vi "Text control 2 v5.3_pump-specific.vi"() -> ()   [LabVIEW 2016]
panel:
  in  "Tab Control":enum32{"Main", "Other parameters"}(tab)
  out "Line running":i32
  out "Total lines":i32
  out "Path":path=path "C:/users/rlp38/09Apr2009LTtesting/test2.txt"
  out "I vs Vg":cluster{"Y data in":dbl[], "X data in":dbl[]}[](graph)
  out "Is max":dbl format="%.2e"
  out "Id max":dbl format="%.2e"
  out "Ig max":dbl format="%.2e"
  out "Imax vs time":cluster{"Y data in":dbl[], "X data in":dbl[]}[](graph)
  out "Imin vs time":cluster{"Y data in":dbl[], "X data in":dbl[]}[](graph)
  out "I vs Vd":cluster{"Y data in":dbl[], "X data in":dbl[]}[](graph)
  in  "Script":string="#-------------------------------------------------------\n# Priming script\n#\n# Version 0.7\n# Author: Dimitrios Simatos\n# Last updated: 2017-10-22\n#-------------------------------------------------------\n# Description\n#\n# This script is designed to prime inlet ports 3, 5 and outlet port 2.\n#-------------------------------------------------------\n# Changes\n#\n# Changed drawing flow to 100 pulses/second.\n#-------------------------------------------------------\n# Important points\n#\n# Never leave any liquid in the pump to dry after the experiments. If they dry, the residue may block the valve.\n# Always run the cleaning cycle after the experiments.\n# Use clockwise rotation when going up in valve port numbers and vice versa.\n#-------------------------------------------------------\n# Things to do before running the script\n#\n# Set time units to minutes.\n# Set filenames.\n# Replace the tubing, if necessary.\n#-------------------------------------------------------\n# Port connections\n#\n# Port 1: Waste\n# Port 2: Waste\n# Port 3: Ultrapure water\n# Port 4: Nothing\n# Port 5: Phosphate buffer (pH=3.2 - 50 mM)\n# Port 6: Nothing\n#-------------------------------------------------------\n# Pumping cycles and execution time\n#\n# Execution time: 4 x 2 = 8 minutes\n# Ultrapure water must be the last to be pumped through the valve, to wash away residual ions.\n# There are 4 pumping cycles. The first two are small, priming cycles, and the last two are large, cleaning and priming cycles.\n# Each small pumping cycle primes the tubing of each port.\n# The last two cycle prime the tubing of the port containing ultrapure water (port 3) and also pump it through the valve, to clean the valve, the syringe, and prime the tubing of the device port (port 2).\n# The device must be disconnected from the port during the priming procedure.\n#-------------------------------------------------------\n# Volume of liquid needed\n#\n# Volume of liquid needed per small cycle: 200 ul\n# Volume of liquid needed per large cycle: 800 ul\n# Total volume of liquid needed per script run:\n# 200 ul of phosphate buffer (pH=3.2 - 50 mM)\n# 200 + 2 x 800 = 1800 ul of ultrapure water\n#-------------------------------------------------------\n# Parameters\n#\n# Syringe size: 1 ml\n# Step resolution N = 0.01 mm\n# Drawing flow V = 100 pulses/second (2000 ul/min)\n# Pumping flow V = 100 pulses/second (2000 ul/min)\n#-------------------------------------------------------\n# Cycle 1: Priming the tubing of port 5\npump /1ZR #initialize pump\npump /1Q #query pump\npump /1? #report absolute plunger position\n#pump /1?6 #report valve position\nwait-min 1 #wait 1 minute\npump /1N0R #set step resolution: 0.01 mm\npump /1Q #query pump\npump /1? #report absolute plunger position (the plunger should be at 0)\npump /1?6 #report valve position\nwait 1000 #wait 1 second\npump /1V100R #choose speed: 100 steps/s (200 ul/min)\npump /1Q #query pump\nwait 1000 #wait 1 second\npump /1O5R #go to port 5, counterclockwise rotation\npump /1Q #query pump\npump /1?6 #report valve position\nwait 1000 #wait 1 second\npump /1A600R #go to absolute position 600 (= draw 200 ul)\n# The position of the plunger depends on the volume of the tubing. The syringe must draw enough liquid to fill the tubing.\nwait 30000 #wait 30 seconds\npump /1Q #query pump\npump /1? #report absolute plunger position (the plunger should have finished moving)\n#pump /1?6 #report valve position\npump /1I1R #switch to port 1, clockwise rotation\npump /1Q #query pump\npump /1?6 #report valve position\npump /1A0R #go to absolute position 0 (= empty syringe)\npump /1Q #query pump\npump /1? #report absolute plunger position (the plunger should be moving to 0)\n#pump /1?6 #report valve position\nwait-min 1 #wait 1 minute\n#-------------------------------------------------------\n# Cycle 2: Priming the tubing of port 3\n#pump /1ZR #initialize pump\npump /1Q #query pump\npump /1? #report absolute plunger position\npump /1?6 #report valve position\nwait-min 1 #wait 1 minute\npump /1N0R #set step resolution: 0.01 mm\npump /1Q #query pump\npump /1? #report absolute plunger position (the plunger should be at 0)\npump /1?6 #report valve position\nwait 1000 #wait 1 second\npump /1V100R #choose speed: 100 steps/s (200 ul/min)\npump /1Q #query pump\nwait 1000 #wait 1 second\npump /1I3R #go to port 3, clockwise rotation\npump /1Q #query pump\npump /1?6 #report valve position\nwait 1000 #wait 1 second\npump /1A600R #go to absolute position 600 (= draw 200 ul)\n# The position of the plunger depends on the volume of the tubing. The syringe must draw enough liquid to fill the tubing.\nwait 30000 #wait 30 seconds\npump /1Q #query pump\npump /1? #report absolute plunger position (the plunger should have finished moving)\n#pump /1?6 #report valve position\npump /1O1R #switch to port 1, counterclockwise rotation\npump /1Q #query pump\npump /1?6 #report valve position\npump /1A0R #go to absolute position 0 (= empty syringe)\npump /1Q #query pump\npump /1?6 #report valve position\npump /1? #report absolute plunger position (the plunger should be moving to 0)\n#pump /1?6 #report valve position\nwait-min 1 #wait 1 minute\n#-------------------------------------------------------\n# Cycle 3: Cleaning the syringe and the tubing of port 2 (1/2)\n#pump /1ZR #initialize pump\npump /1Q #query pump\npump /1? #report absolute plunger position\npump /1?6 #report valve position\nwait-min 1 #wait 1 minute\npump /1N0R #set step resolution: 0.01 mm\npump /1Q #query pump\npump /1? #report absolute plunger position (the plunger should be at 0)\npump /1?6 #report valve position\nwait 1000 #wait 1 second\npump /1V100R #choose speed: 100 steps/s (200 ul/min)\npump /1Q #query pump\nwait 1000 #wait 1 second\npump /1I3R #go to port 3, clockwise rotation\npump /1Q #query pump\npump /1?6 #report valve position\nwait 1000 #wait 1 second\npump /1A2400R #go to absolute position 2400 (= draw 800 ul)\n# The position of the plunger depends on the volume of the tubing. The syringe must draw enough liquid to fill the tubing.\nwait 30000 #wait 30 seconds\npump /1Q #query pump\npump /1? #report absolute plunger position (the plunger should have finished moving)\n#pump /1?6 #report valve position\npump /1O2R #switch to port 2, counterclockwise rotation\npump /1Q #query pump\npump /1?6 #report valve position\npump /1A0R #go to absolute position 0 (= empty syringe)\npump /1Q #query pump\npump /1? #report absolute plunger position (the plunger should be moving to 0)\n#pump /1?6 #report valve position\nwait-min 1 #wait 1 minute\n#-------------------------------------------------------\n# Cycle 4: Cleaning the syringe and the tubing of port 2 (2/2)\n#pump /1ZR #initialize pump\npump /1Q #query pump\npump /1? #report absolute plunger position\npump /1?6 #report valve position\nwait-min 1 #wait 1 minute\npump /1N0R #set step resolution: 0.01 mm\npump /1Q #query pump\npump /1? #report absolute plunger position (the plunger should be at 0)\npump /1?6 #report valve position\nwait 1000 #wait 1 second\npump /1V100R #choose speed: 100 steps/s (200 ul/min)\npump /1Q #query pump\nwait 1000 #wait 1 second\npump /1I3R #go to port 3, clockwise rotation\npump /1Q #query pump\npump /1?6 #report valve position\nwait 1000 #wait 1 second\npump /1A2400R #go to absolute position 2400 (= draw 800 ul)\n# The position of the plunger depends on the volume of the tubing. The syringe must draw enough liquid to fill the tubing.\nwait 30000 #wait 30 seconds\npump /1Q #query pump\npump /1? #report absolute plunger position (the plunger should have finished moving)\n#pump /1?6 #report valve position\npump /1O2R #switch to port 2, counterclockwise rotation\npump /1Q #query pump\npump /1?6 #report valve position\npump /1A0R #go to absolute position 0 (= empty syringe)\npump /1Q #query pump\npump /1? #report absolute plunger position (the plunger should be moving to 0)\n#pump /1?6 #report valve position\nwait-min 1 #wait 1 minute\n#-------------------------------------------------------"
  out "Command running:":string
  out "Serial port data":string
  out "Elapsed Time":dbl caption="Elapsed Time (s)"
  in  "Units":u16(ring)=1 items=["Seconds", "Minutes", "Hours"]
  in  "Time Offset":dbl caption="Set Start Time (s)"
  in  "Reset":bool
  in  "Auto Reset":bool
  in  "integration time":u32(slide) max=2 step=1 scale=0.0..2.0
  in  "Interrupt run":bool
  out "Absolute plunger position vs time":cluster{"Y data in":dbl[], "X data in":dbl[]}[](graph)
  out "Valve position vs time":cluster{"Y data in":dbl[], "X data in":dbl[]}[](graph)
  in  "Halt pump":bool
  in  "Hard stop pump":bool
  out "Is on":dbl format="%.2e"
  out "Id on":dbl format="%.2e"
  out "Ig on":dbl format="%.2e"
  out "Ion vs time":cluster{"Y data in":dbl[], "X data in":dbl[]}[](graph)
  out "Ioff vs time":cluster{"Y data in":dbl[], "X data in":dbl[]}[](graph)
  out "Ig min":dbl format="%.2e"
  out "Id min":dbl format="%.2e"
  out "Is min":dbl format="%.2e"
  out "Is off":dbl format="%.2e"
  out "Id off":dbl format="%.2e"
  out "Ig off":dbl format="%.2e"
  in  "Gate Range\nmode":u16(ring) items=["Auto", "Limited", "Fixed"]
  in  "Gate Range":u8(slide)=6 max=11 scale=0.0..11.0
  in  "Source/Drain\nRange mode":u16(ring) items=["Auto", "Limited", "Fixed"]
  in  "Source/Drain Range":u8(slide)=6 max=11 scale=0.0..11.0
  in  "Panel Controls":T1={"Emergency Stop"=refnum, "TransGraph Max"=1e-05, "Text/Graph (text=false)"=TRUE} {"TransGraph Max" format="%.2e"}
  in  "Panel Controls 2":T2={"Emergency Stop"=refnum, "TransGraph Max"=1e-05, "Text/Graph (text=false)"=TRUE, "TransGraph Min"=1e-11} {"TransGraph Min" format="%.2e"; "TransGraph Max" format="%.2e"}
  in  "SMU4":cluster{"on/off":bool, "Voltage":dbl} {"Voltage" min=-100.0 max=100.0 format="%.2f"}
  in  "Full Reset":bool
  in  "Standby":T3
  out "error out":errorcluster
  in  "Delay before read (ms)":u32=1000
  in  "byte count":u32=64
  in  "Serial End Mode for Reads":u16(ring)=2 items=["None", "LastBit", "TermChar"]
  in  "Timeout (ms)":u32=10000
  in  "Enable Termination\nChar (T)":bool=TRUE
  in  "Termination char\n(0xA = '\\n' = LF)\n(0xD = '\\r' = CR)":u8=13 format="%.0x"
  in  "flow control":u16(ring) items=["None"=0, "XON/XOFF"=1, "RTS/CTS"=2, "DTR/DSR"=4]
  in  "stop bits":u16(ring)=10 items=["1.0"=10, "1.5"=15, "2.0"=20]
  in  "parity":u16(ring) items=["None", "Odd", "Even", "Mark", "Space"]
  in  "data bits":u16=8 min=5 max=8 step=1
  in  "VISA resource name":refnum<visa-resource-name>="COM6"
  in  "baud rate":u32=9600
  in  "Drain: Compliance":dbl=0.001 format="%.8f"
  in  "Gate: Compliance":dbl=0.001 format="%.8f"
  in  "hold time /s":dbl format="%.2f"
  in  "delay time /s":dbl format="%.2f"
  in  "Integration time (short)":dbl=0.0019 min=8e-05 max=0.0019 step=8e-05 format="%^.0e"
  in  "Integration time (long)":dbl=0.32 min=0.04 max=2.0 step=0.02 format="%.2f"
  in  "Step delay /s":dbl format="%.2f"
  in  "Filename (variable part)":string="step_1_ultrapure_H2O_"
  in  "Suffix (script)":string="step_1_ultrapure_H2O_script.txt"
  in  "Gate":T4={"Gate Start"=0.0, "Gate Stop"=2.0, "Gate Step (linear only)"=1.0, "Gate Compliance"=0.0001, "Gate PComp"=0.0, "Range mode"=0, "Range"=6} {"Range" max=11 scale=0.0..11.0; "Range mode" items=["Auto", "Limited", "Fixed"]; "Gate PComp" format="%^.2e"; "Gate Compliance" format="%^.2e"; "Gate Step (linear only)" format="%^.4e"; "Gate Stop" format="%^.4e"; "Gate Start" format="%^.4e"}
  in  "Drain 2":T5={"Drain Start"=0.0, "Drain Stop"=2.0, "Drain Compliance"=0.0001, "Drain Step"=1.0, "Drain PComp"=0.0, "Range mode"=0, "Range"=6} {"Range" max=11 scale=0.0..11.0; "Range mode" items=["Auto", "Limited", "Fixed"]; "Drain PComp" format="%^.2e"; "Drain Step" format="%^.4e"; "Drain Compliance" format="%^.2e"; "Drain Stop" format="%^.4e"; "Drain Start" format="%^.4e"}
  in  "Timings 2":T6={"integration time"=0, "Short/Long integration time"=0.00064, "hold time (sec)"=0.0, "delay time (sec)"=0.0, "Step Time (0 disables)"=0.0, "sweep method"=0, "Pulse period"=0.005, "Base voltage"=0.0, "Pulse width"=0.0005} {"Pulse width" min=0.0005 max=0.1 step=0.0001 format="%.4f"; "Base voltage" format="%^.4e"; "Pulse period" min=0.005 max=1.0 step=0.0001 format="%.4f"; "sweep method" items=["Continuous", "Pulsed"]; "Step Time (0 disables)" format="%.2f"; "delay time (sec)" format="%.4f"; "hold time (sec)" format="%.4f"; "Short/Long integration time" format="%^.0e"; "integration time" scale=0.0..2.0}
  # "Syntax:\nitime [s|m|l]\ngaterangemode [a|l|f]\ndrainrangemode [a|l|f]\npulsed [on|off] PulsePeriod(sec) PulseBaseVoltage PulseONWidth(sec)\nstandby [on l off]\nwait NumMilliseconds\nwait-min NumMinutes\n# texthere = comment\ntransfer [s|d] VgStart VgStop VgStep VdStart VdStop VdStep\noutput [s|d] VgStart VgStop VgStep VdStart VdStop VdStep\nsample Vg Vd NumSamples Time(s) SampleInterval(s)\nsamplei Idg NumSamples Time(s) SampleInterval(s) VDGcompliance\n100 samples is approximately 13 seconds with medium integration\n# if in doubt use SampleInterval(s) = 0.004\nstressV VG VD IGcompliance IDcompliance Duration(sec)\nstressI IDG VDGcompliance Duration(sec)\nvsu2pulse Bias Duration(s)\npulsedstressV [s|d] VEstop VgON VgOFF Period(s) PulseONwidth(s) Vd\nsample-fpp Vg Vd NumSamples Time\nresample-fpp Vg Vd\ntransfer-fpp [s|d] VgStart VgStop VgStep VdStart VdStop VdStep\noutput-fpp [s|d] VgStart VgStop VgStep VdStart VdStop VdStep\nserial SerialPortCommand\npump SerialPortCommand for the SPM pump\n\nSPM Pump Syntax (<x>: pump number, use 1 if only one pump):\nif the command syntax contains [R], then append the letter R to the command\n/<x>Q: query (a query command should follow each command)\n/<x>Z[R] or /<x>Y[R]: initialize pump\n/<x>N<n>[R] (<n>=0,1): <0> (<1>) microstep 0.01 mm (0.00125 mm) resolution\n/<x>I<n> (<n>=0-6): turn to port number n (clockwise)\n/<x>O<n> (<n>=0-6): turn to port number n (counterclockwise)\n/<x>X: Re-execute last command string\n/<x>G<n>[R] (<n>=0-60000): repeat command sequence (default: 0, 0=loop forever)\n/<x>g: Mark the start of a repeat sequence (max = 10)\n/<x>M<n>[R] (<n>=0-86400000): delay command execution by n milliseconds\n/<x>H: Halt; Pause the sequence after finishing the current move\n/<x>T: Hardstop; Interrupt the current move and suppress it from the sequence\n/<x>A<n>[R] (<n>=0-3000 with N=0, 0-24000 with N=1): absolute position\n/<x>P<n>[R] (<n>=0-3000 with N=0, 0-24000 with N=1): relative pickup\n/<x>D<n>[R] (<n>=0-3000 with N=0, 0-24000 with N=1): relative dispense\n/<x>V<n>[R] (<n>=1-1600 default: 150): set peak speed (pulses/sec)\nNOTE: The lowest speed limit is 1 pulse/sec, not 5, as the manual states.\n/<x>S<n>[R] (<n>=10-40 default: 22): set speed (NOT in pulses/sec, look in manual)\nNOTE: When controlled with absolute position, one does not need to pay special attention to the syringe that is mounted on the pump.\nWithdraw from lower stage (ports 3, 5), dispense from higher stage (ports 2, 4, 6).\nConnect Port 1 to waste."
  # "Time"
  # "1\n2\n3\n4\n5\n6\n7\n8\n9\n10\n11\n12\n13\n14\n15\n16\n17\n18\n19\n20"
  # "Serial port settings"
  # "Filename settings"
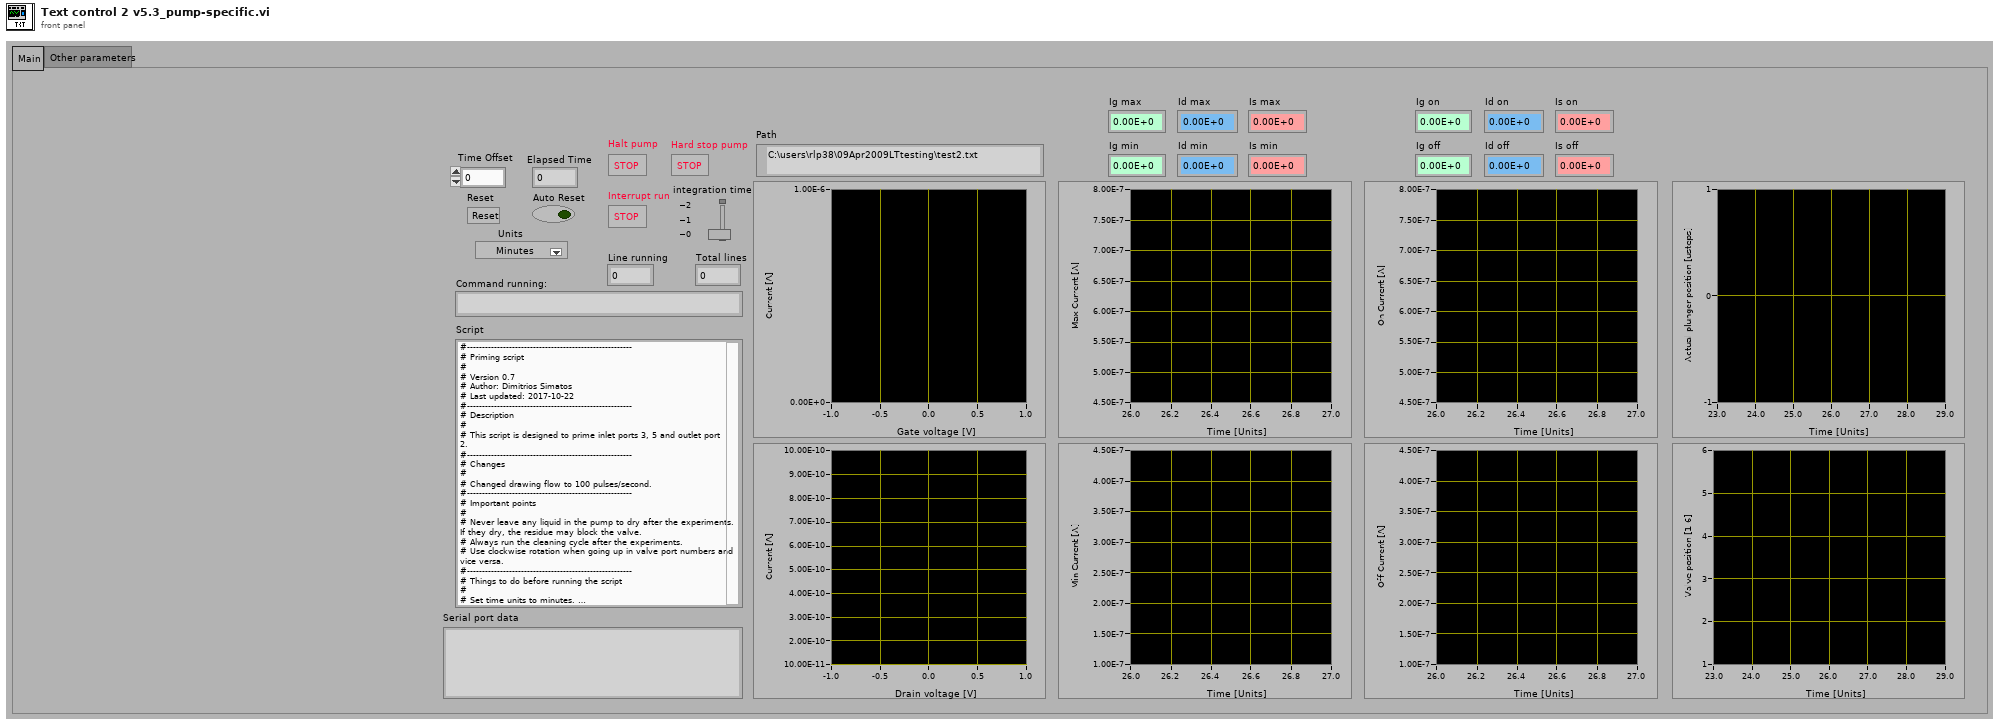
[diagram p1: front panel]
types:
  T1 = cluster{"Emergency Stop":refnum<vi>, "TransGraph Max":dbl, "Text/Graph (text=false)":bool}
  T2 = cluster{"Emergency Stop":refnum<vi>, "TransGraph Max":dbl, "Text/Graph (text=false)":bool, "TransGraph Min":dbl}
  T3 = cluster{"Gate Standby":bool, "Drain Standby":bool}
  T4 = cluster{"Gate Start":dbl, "Gate Stop":dbl, "Gate Step (linear only)":dbl, "Gate Compliance":dbl, "Gate PComp":dbl, "Range mode":u16, "Range":u8}
  T5 = cluster{"Drain Start":dbl, "Drain Stop":dbl, "Drain Compliance":dbl, "Drain Step":dbl, "Drain PComp":dbl, "Range mode":u16, "Range":u8}
  T6 = cluster{"integration time":u32, "Short/Long integration time":dbl, "hold time (sec)":dbl, "delay time (sec)":dbl, "Step Time (0 disables)":dbl, "sweep method":u16, "Pulse period":dbl, "Base voltage":dbl, "Pulse width":dbl}
  T7 = enum16{"open", "replace", "create", "open or create", "replace or create", "replace or create with confirmation"}
  T8 = cluster{"V2 Start":dbl, "V2 Step":dbl, "Number of points":i32}
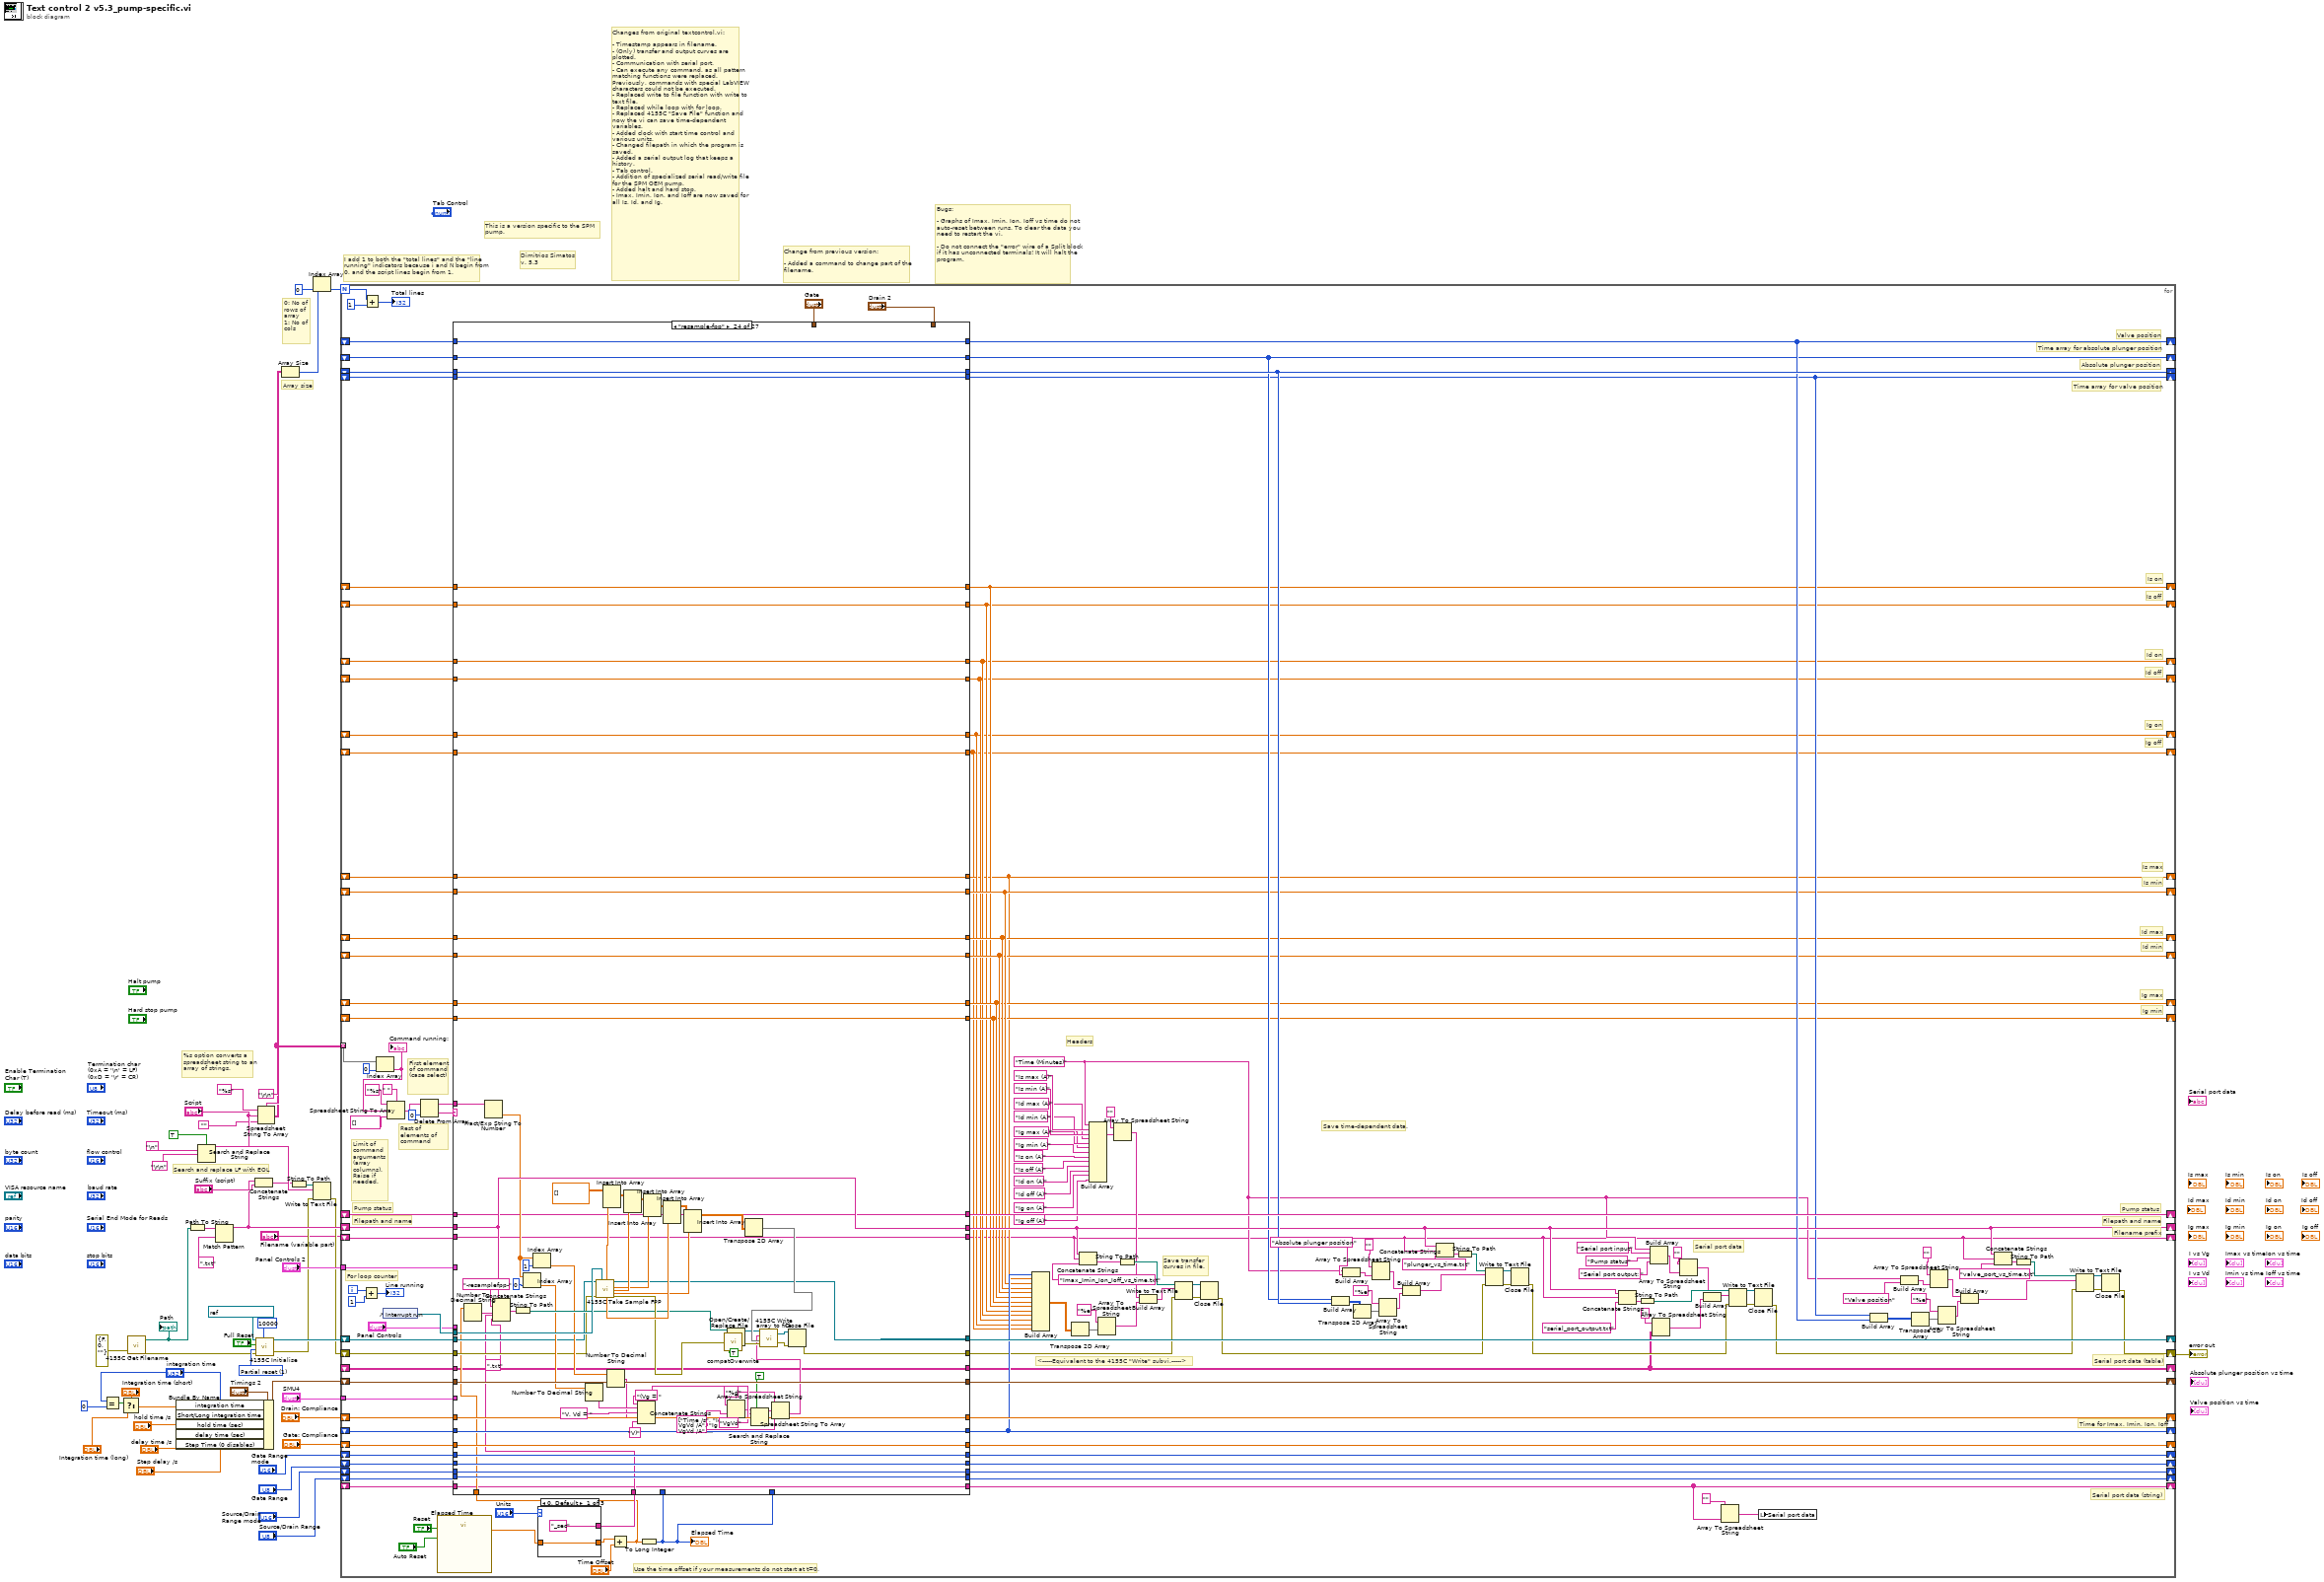
[diagram p0: block diagram]
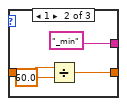
[diagram p2: hidden frame]
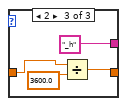
[diagram p3: hidden frame]
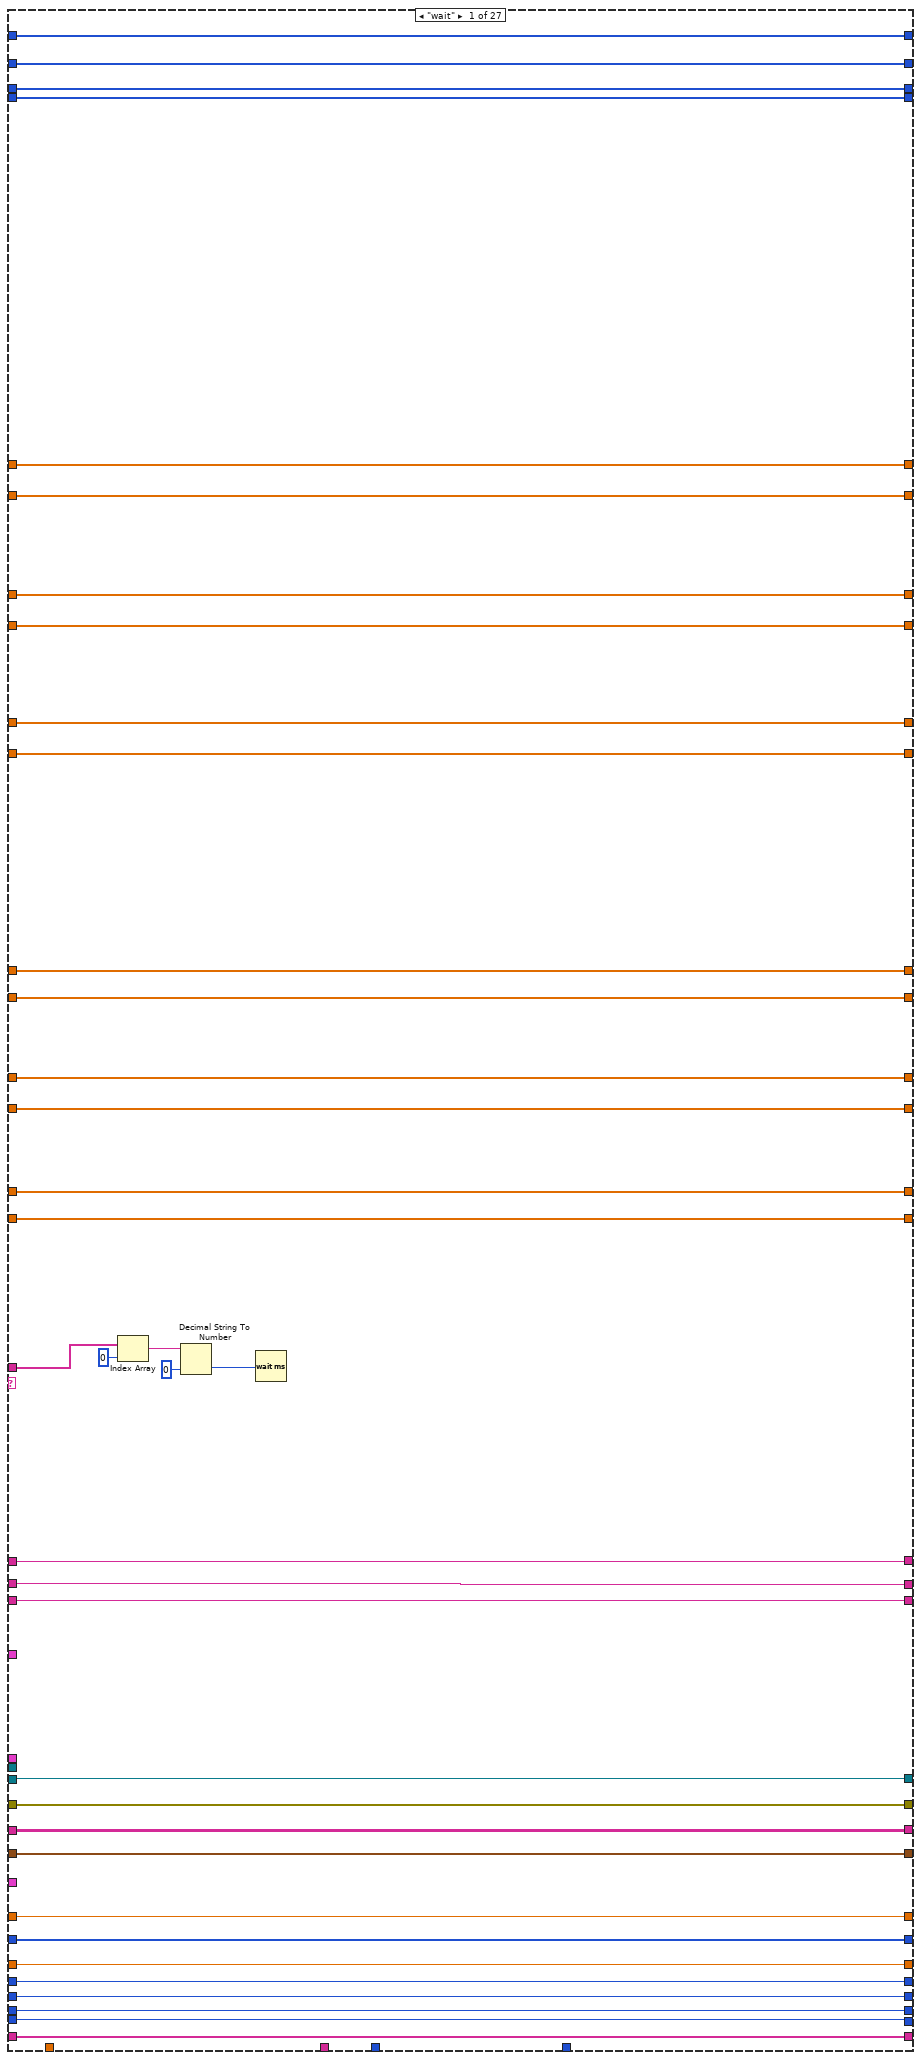
[diagram p4: hidden frame]
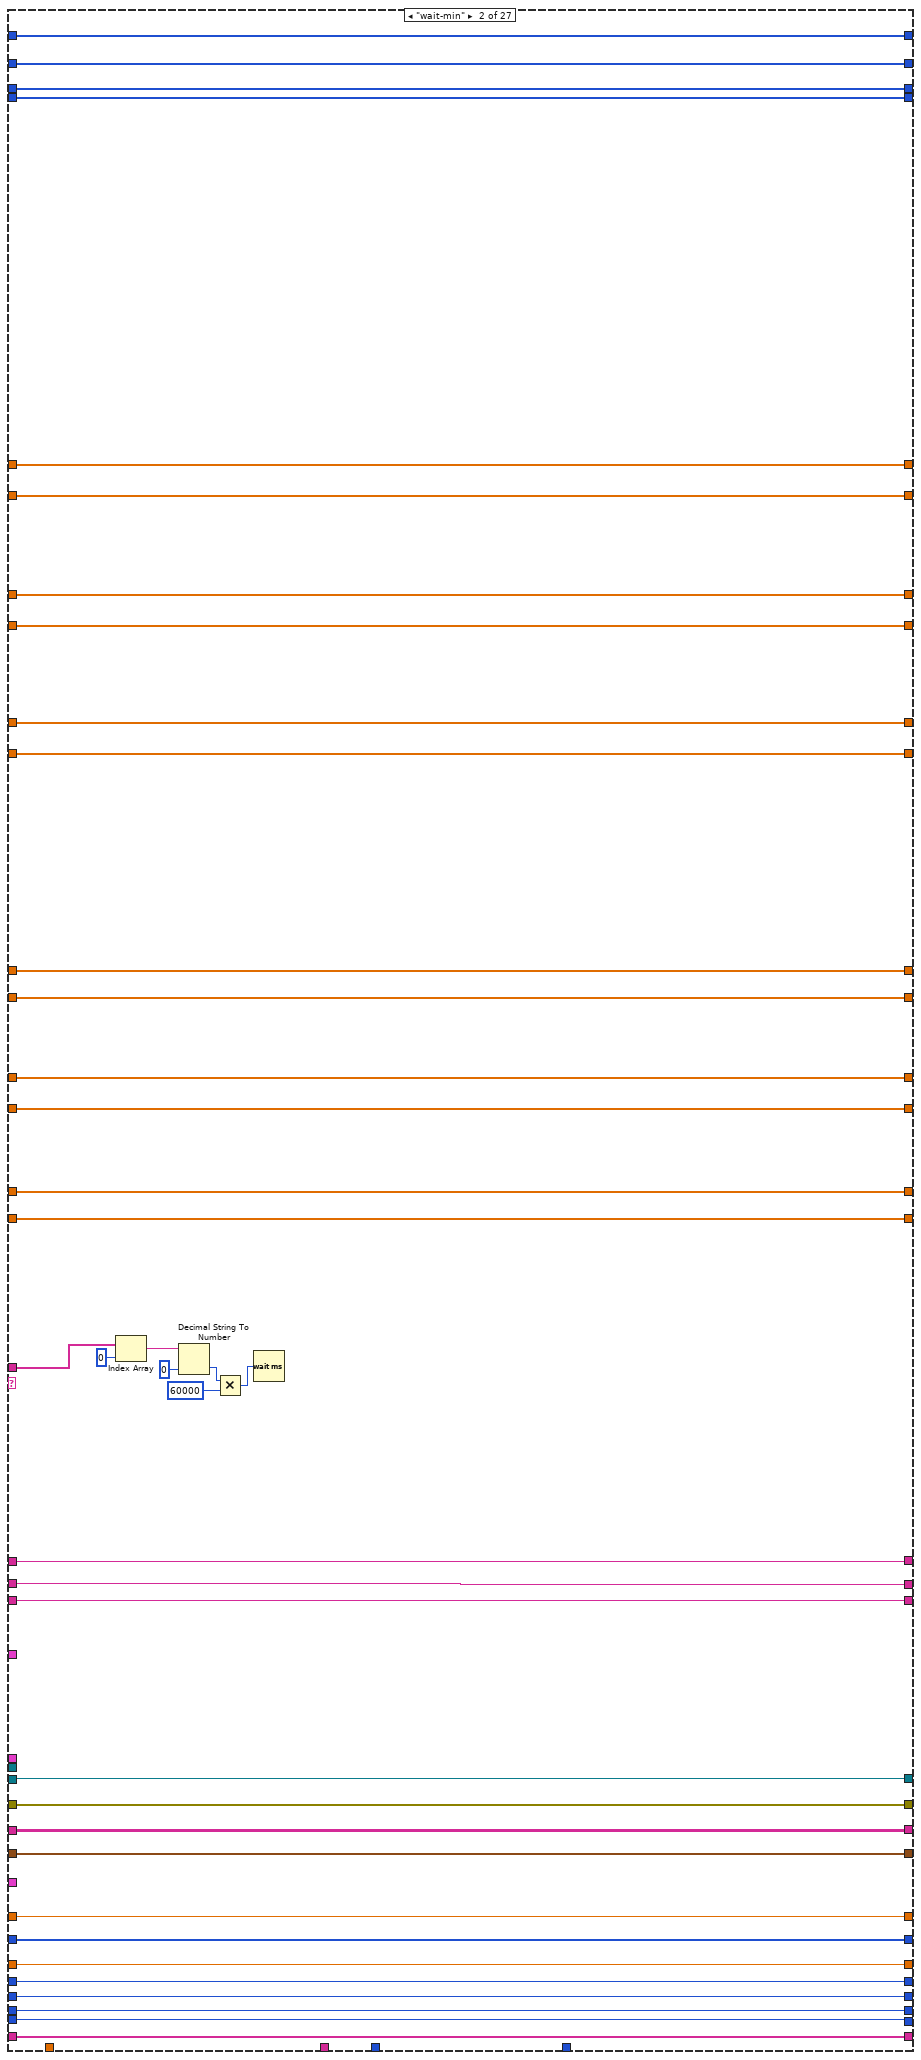
[diagram p5: hidden frame]
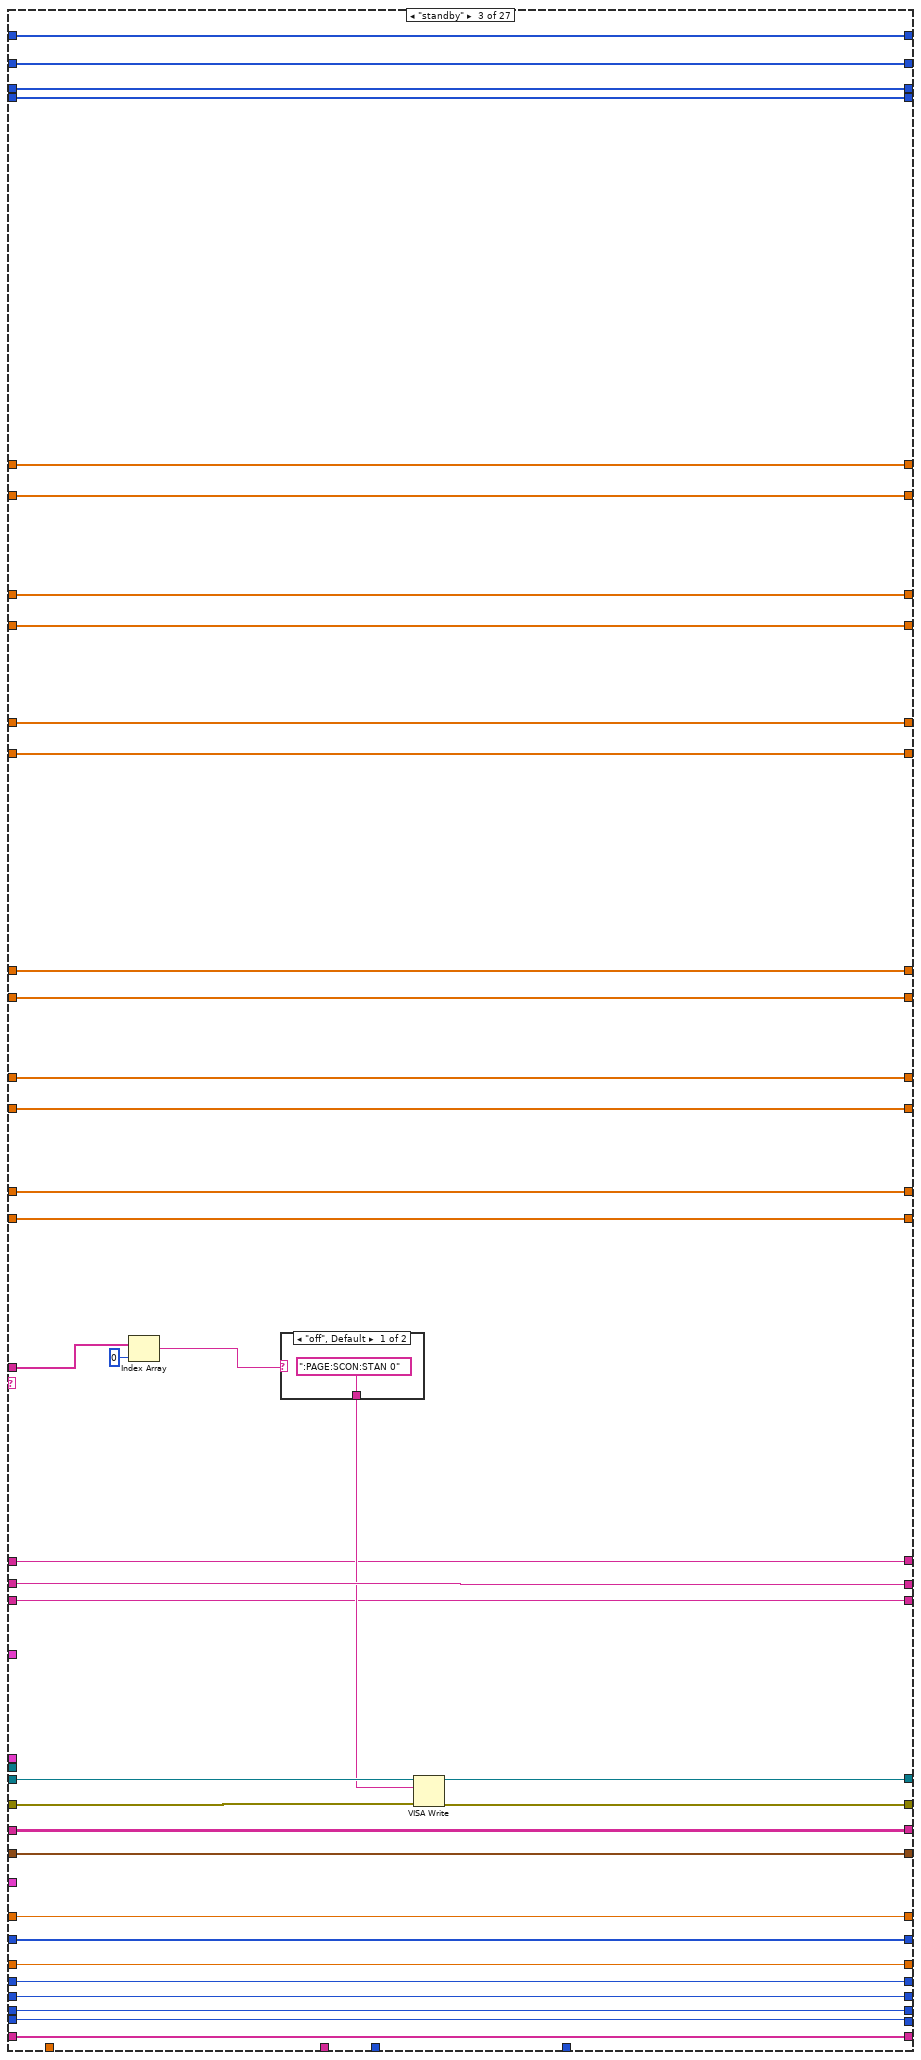
[diagram p6: hidden frame]
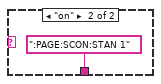
[diagram p7: hidden frame]
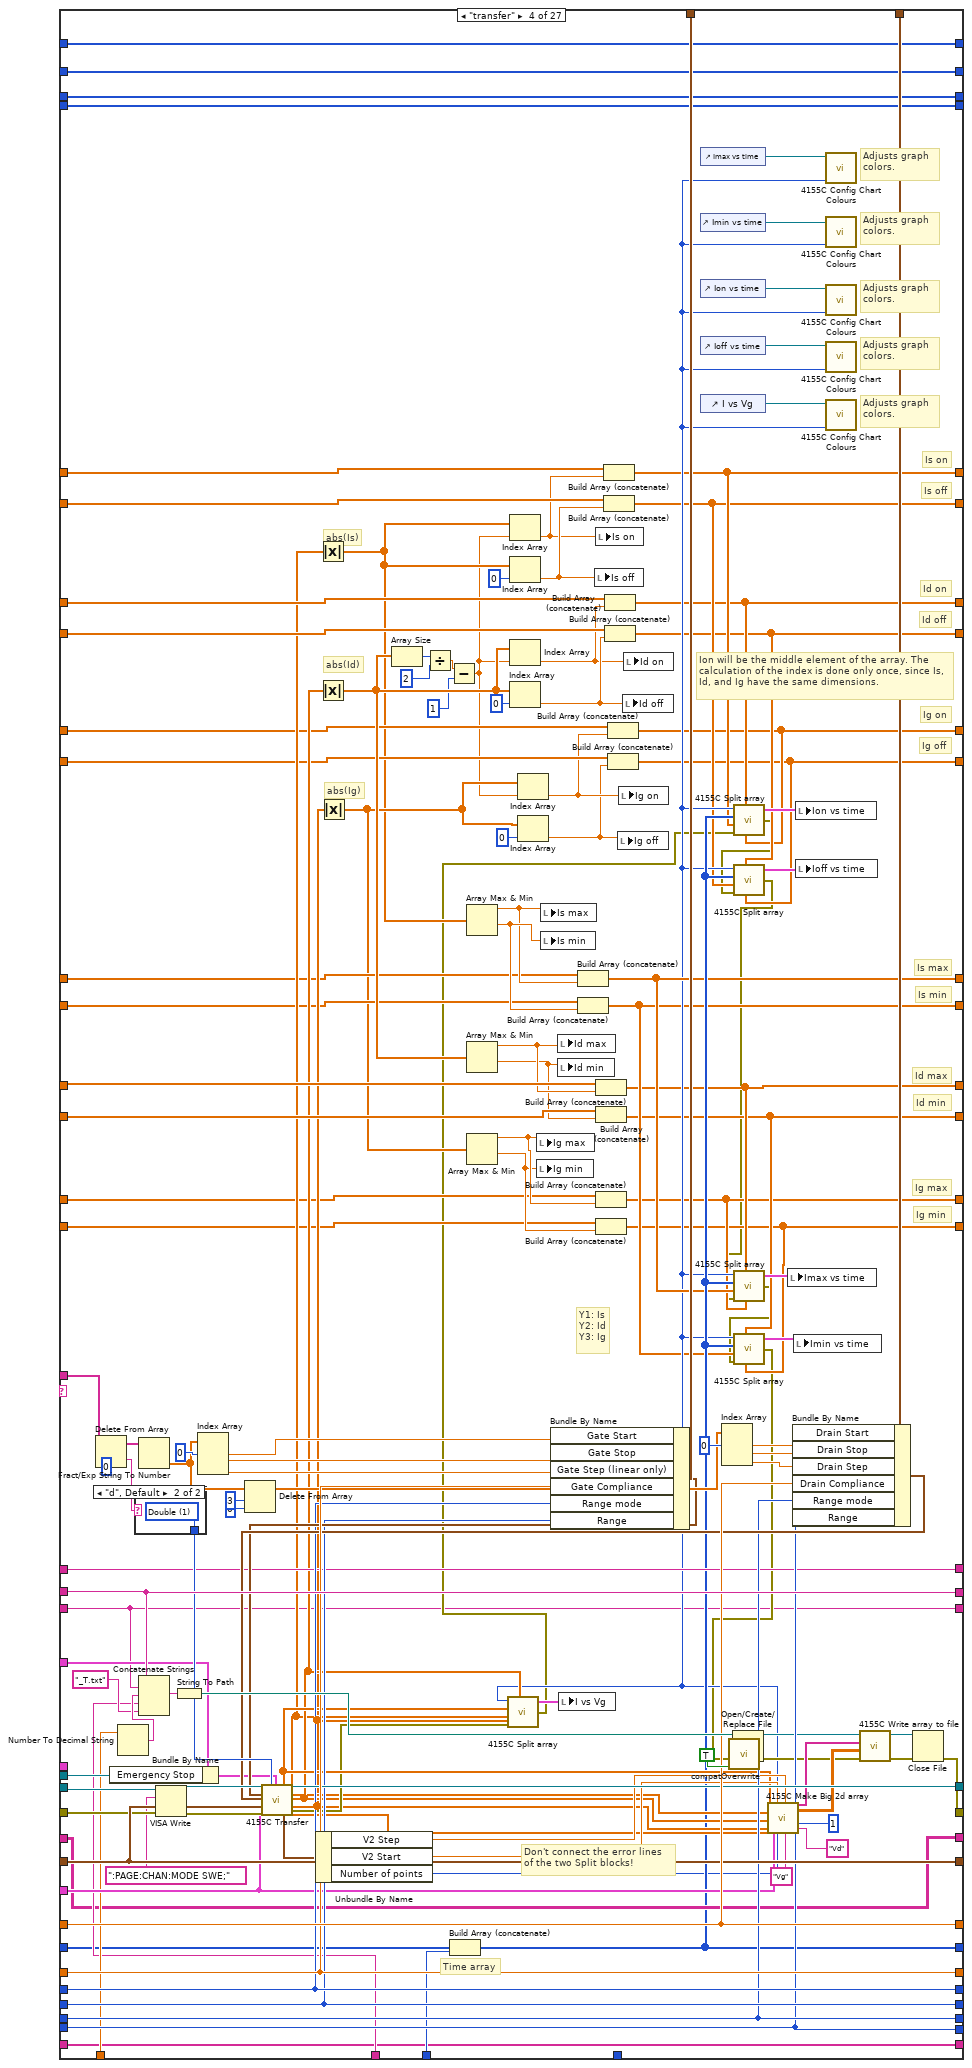
[diagram p8: hidden frame]
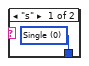
[diagram p9: hidden frame]
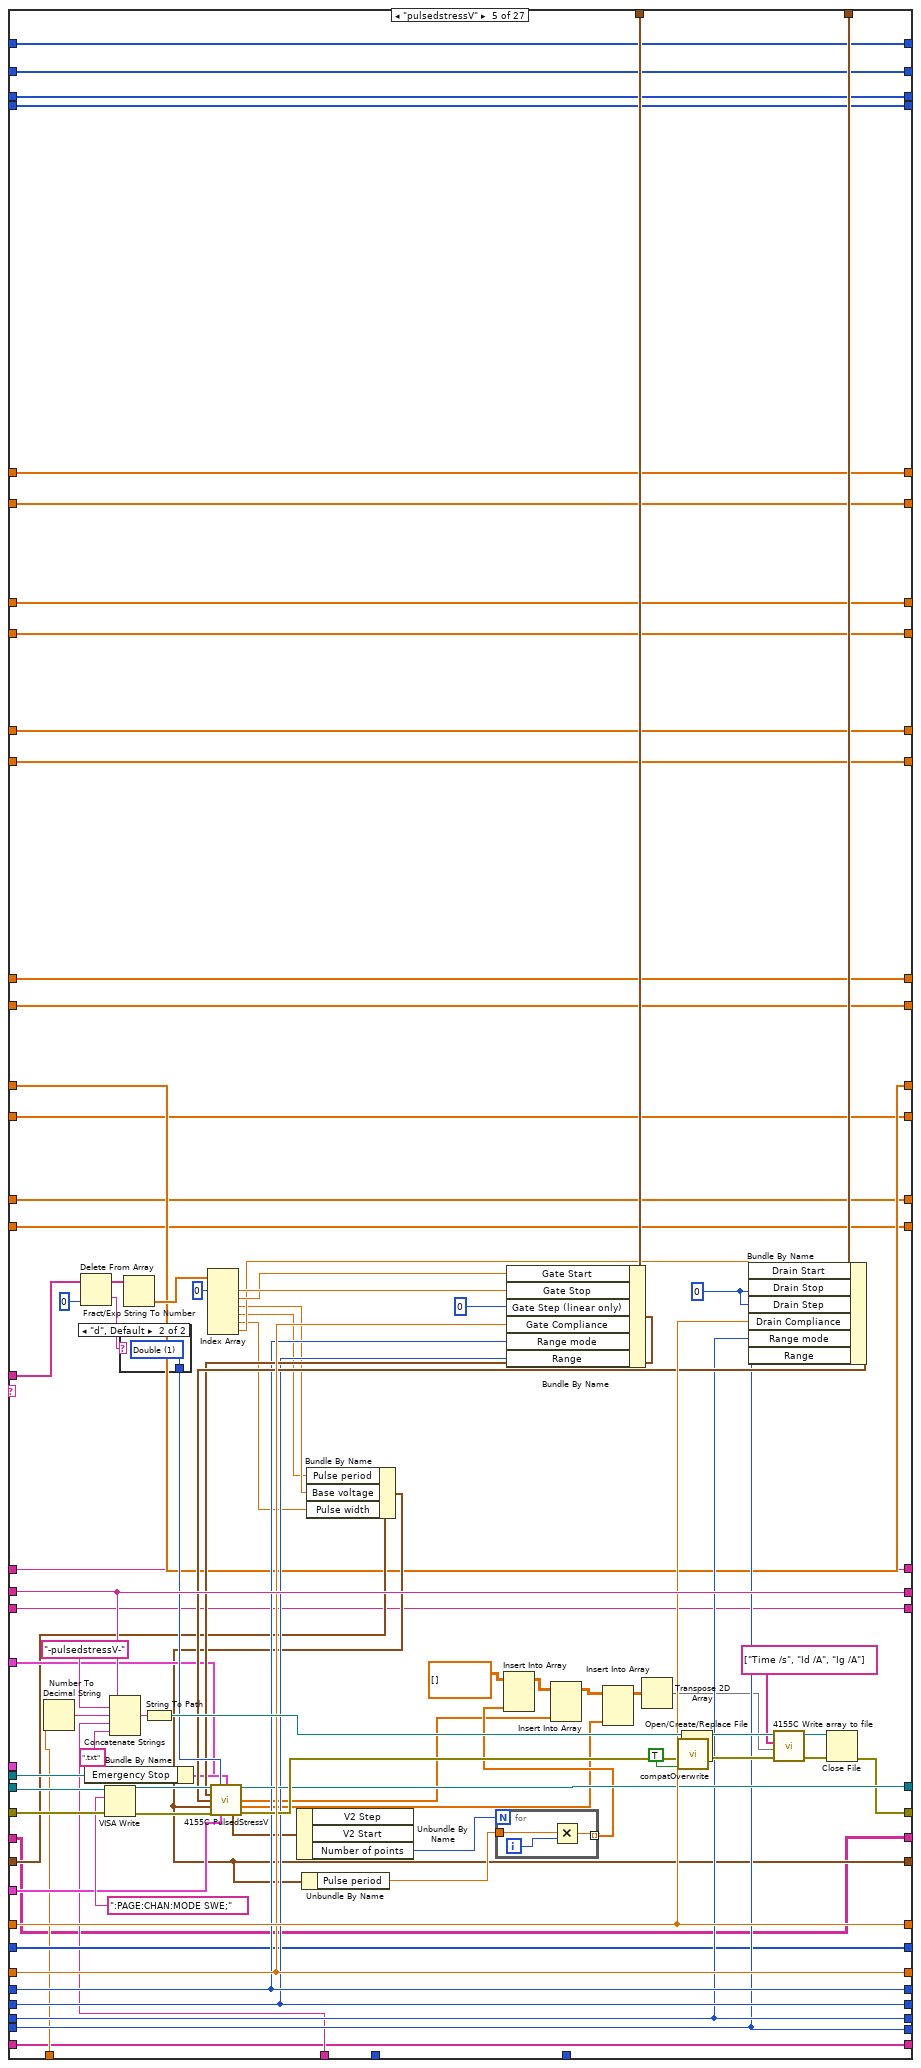
[diagram p10: hidden frame]
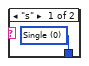
[diagram p11: hidden frame]
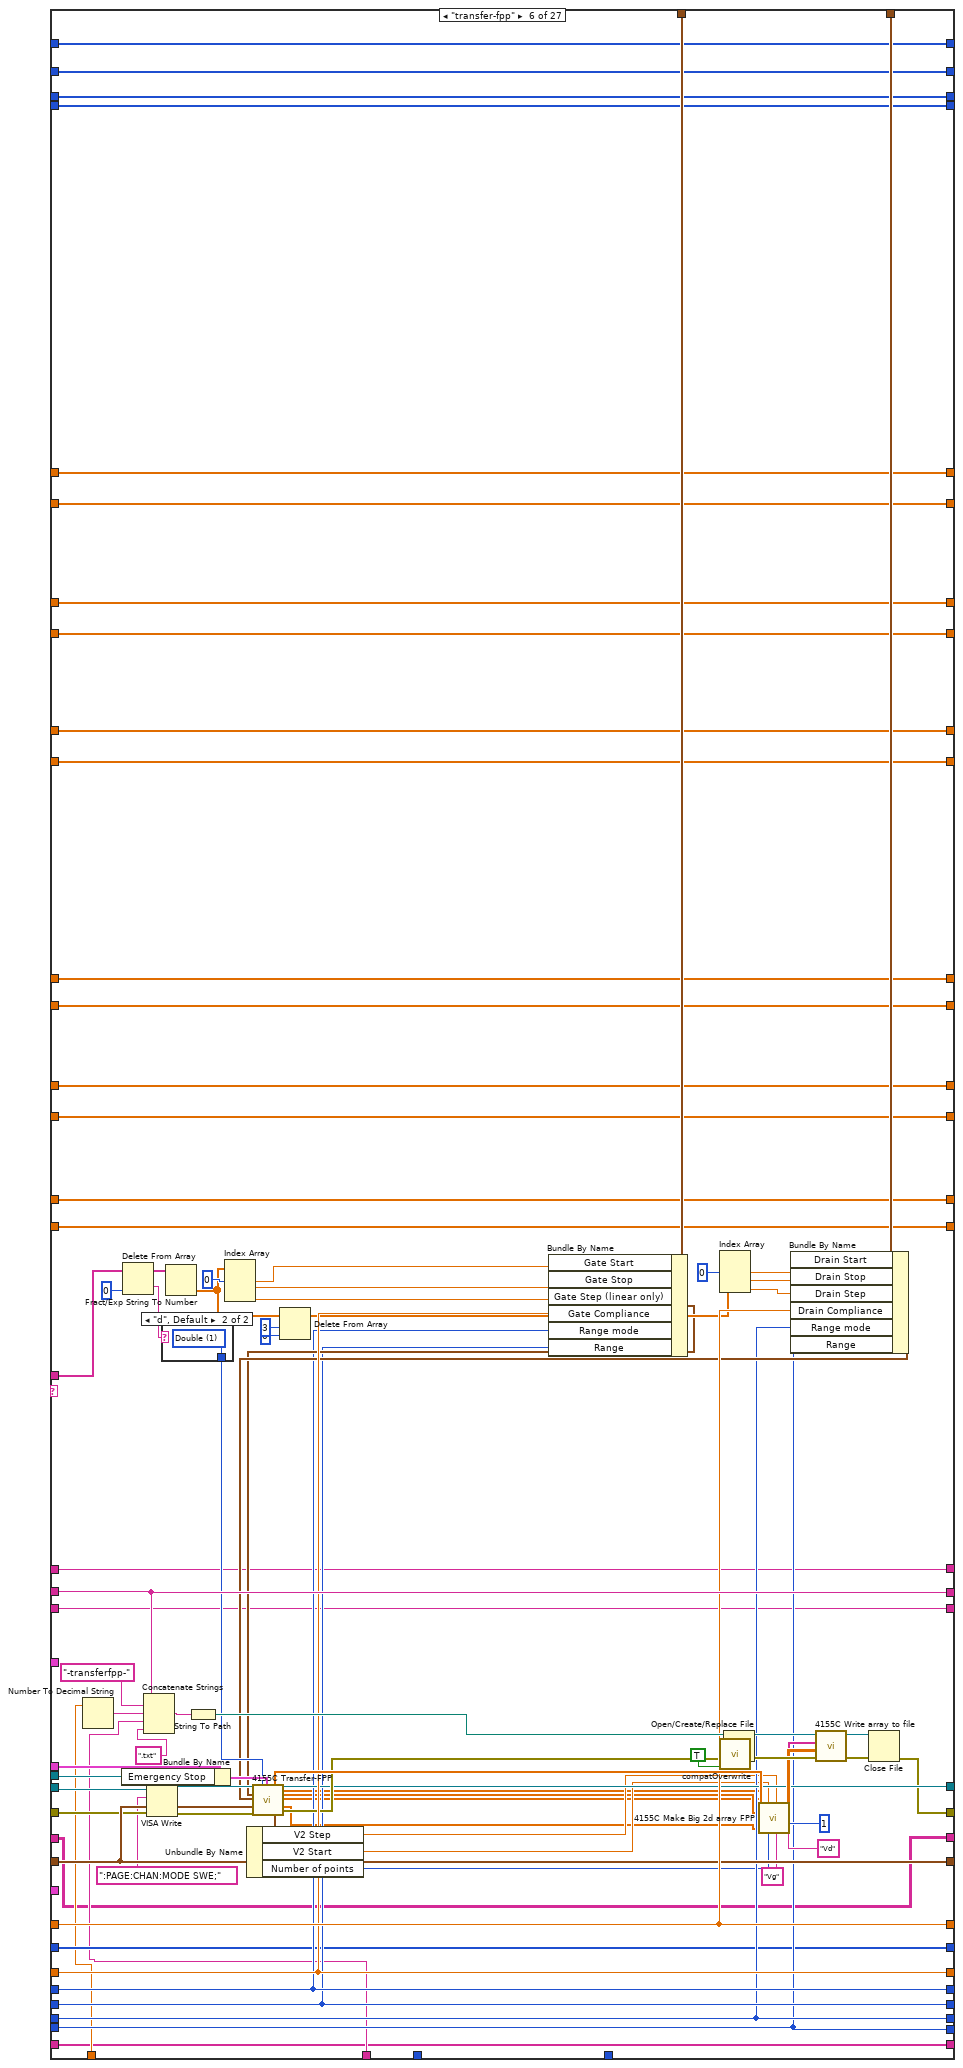
[diagram p12: hidden frame]
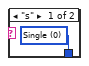
[diagram p13: hidden frame]
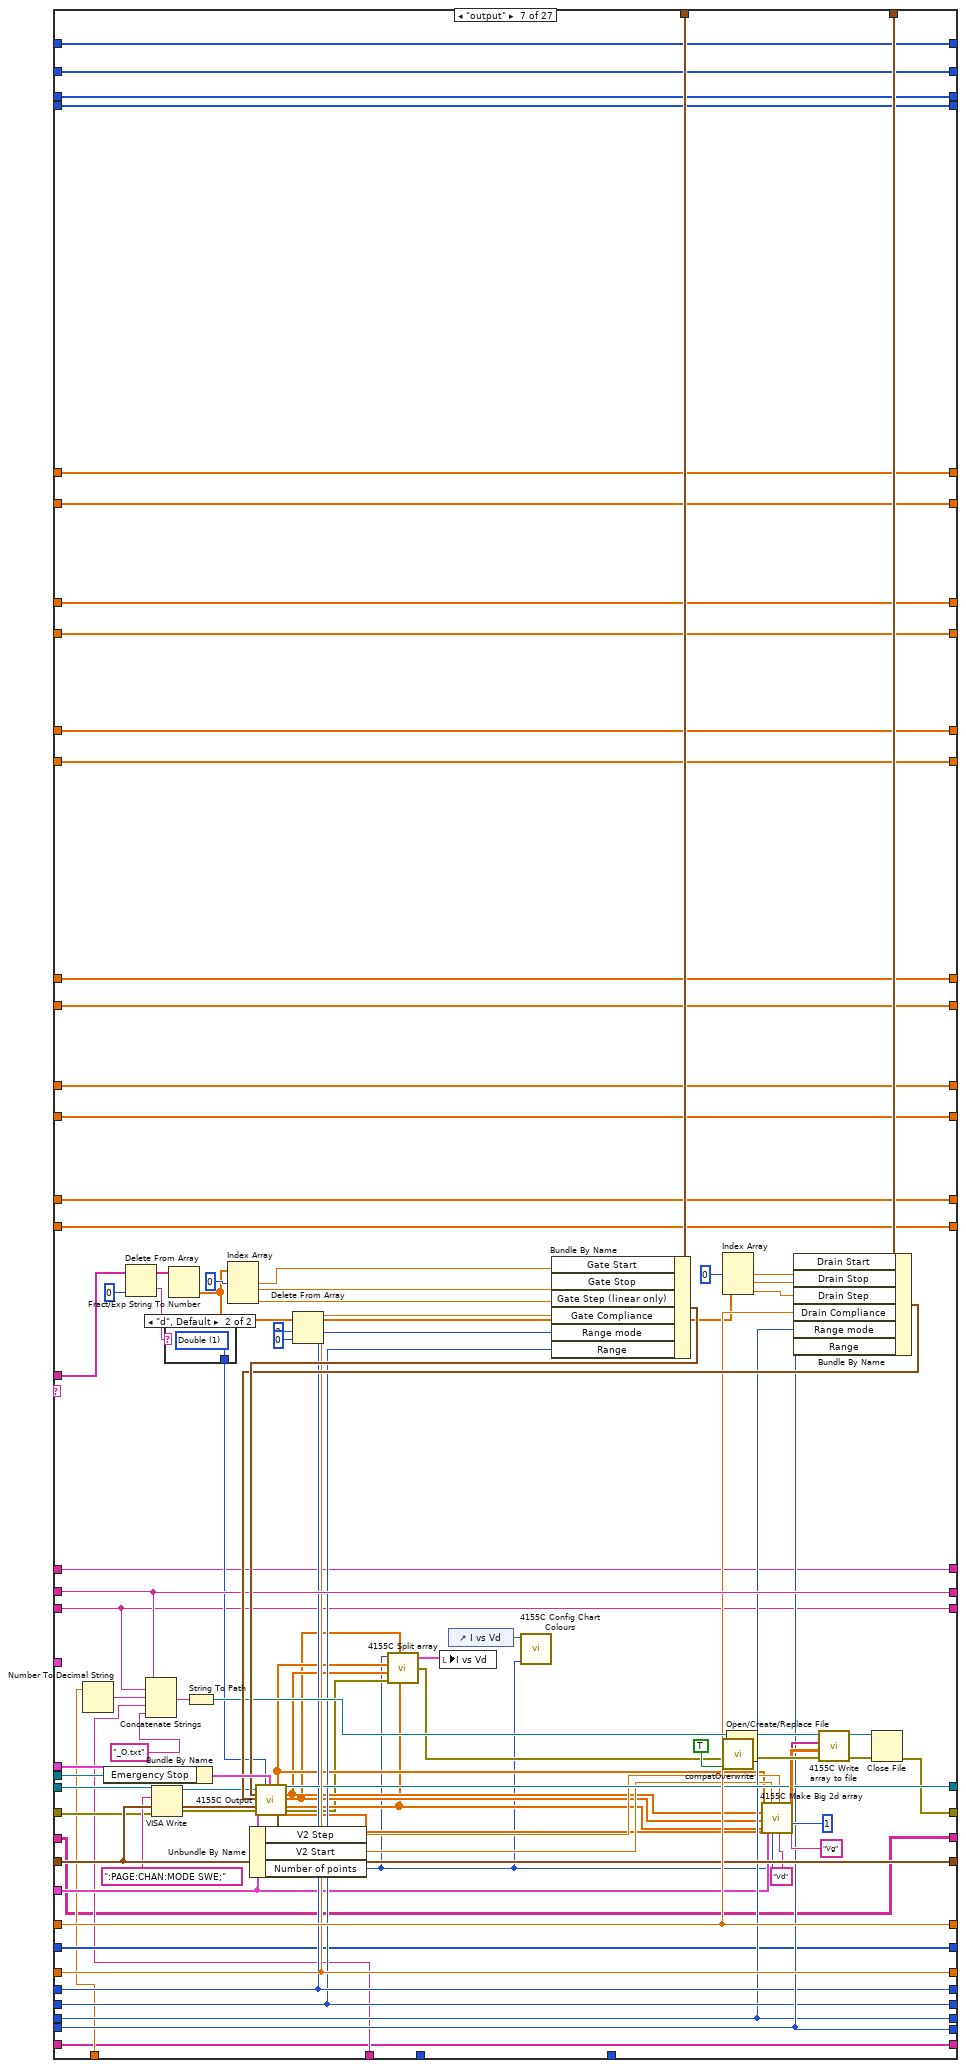
[diagram p14: hidden frame]
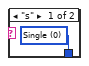
[diagram p15: hidden frame]
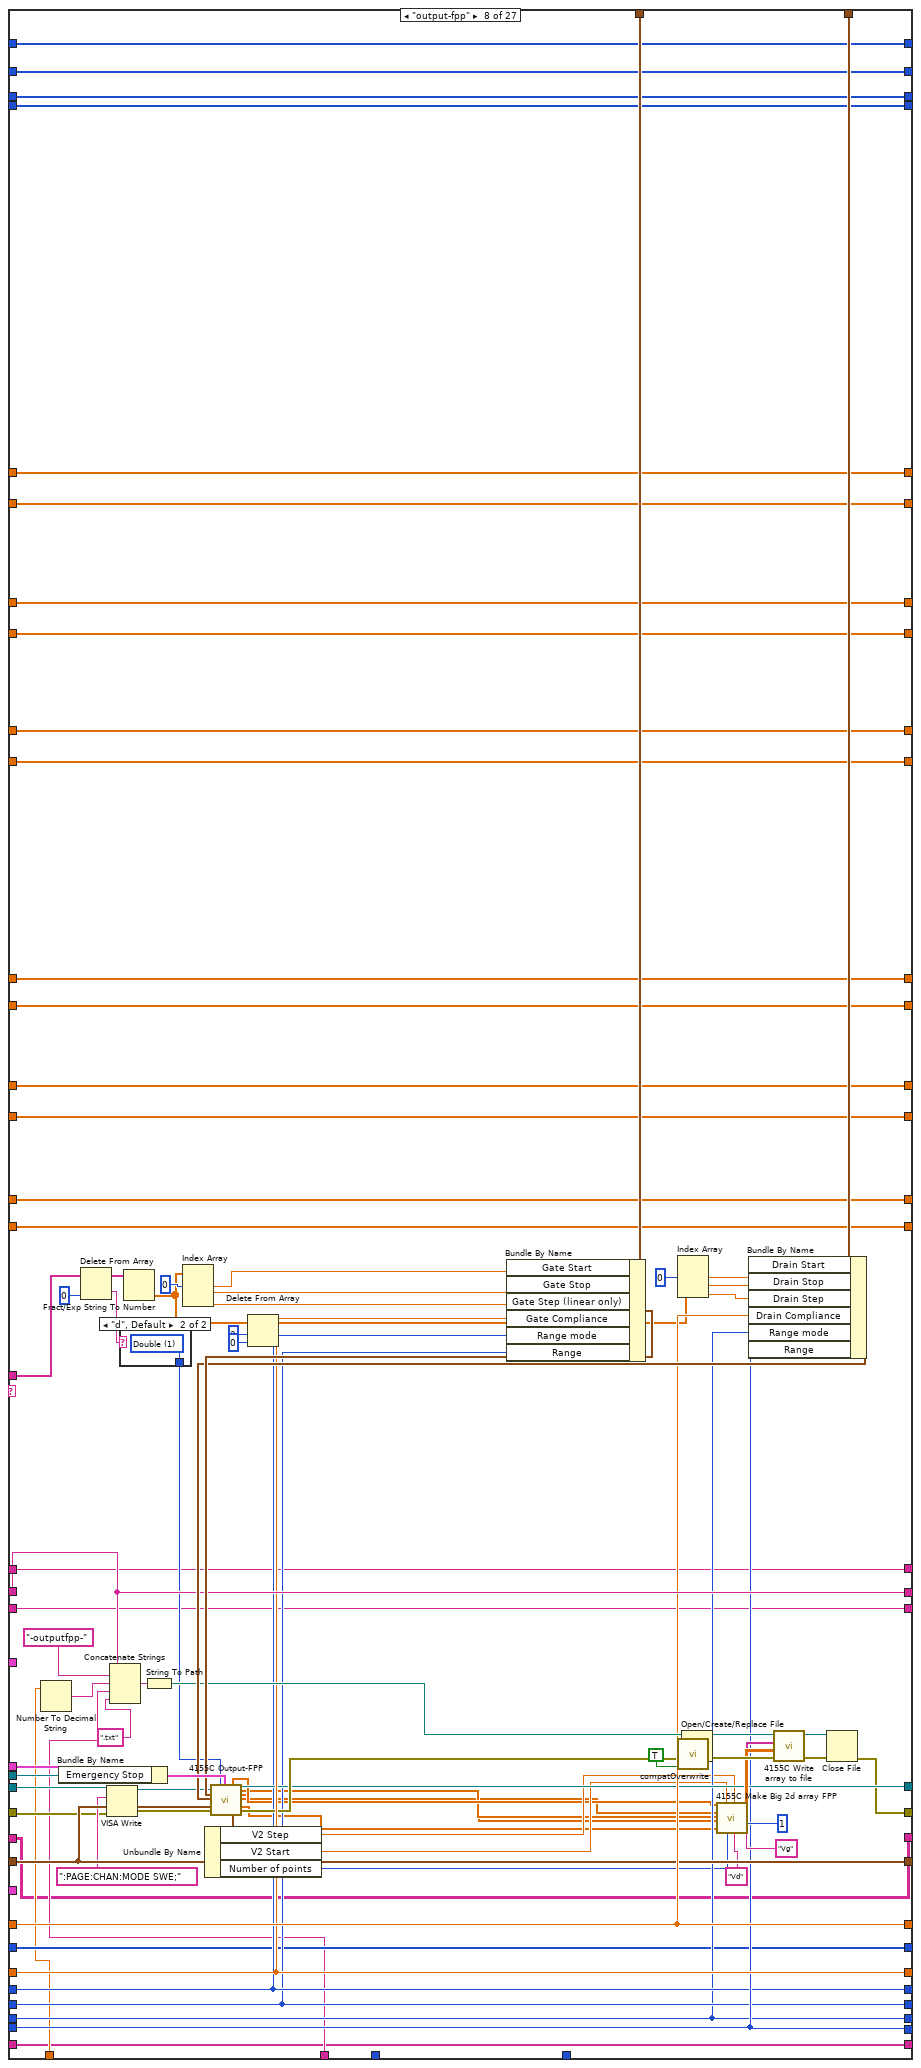
[diagram p16: hidden frame]
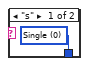
[diagram p17: hidden frame]
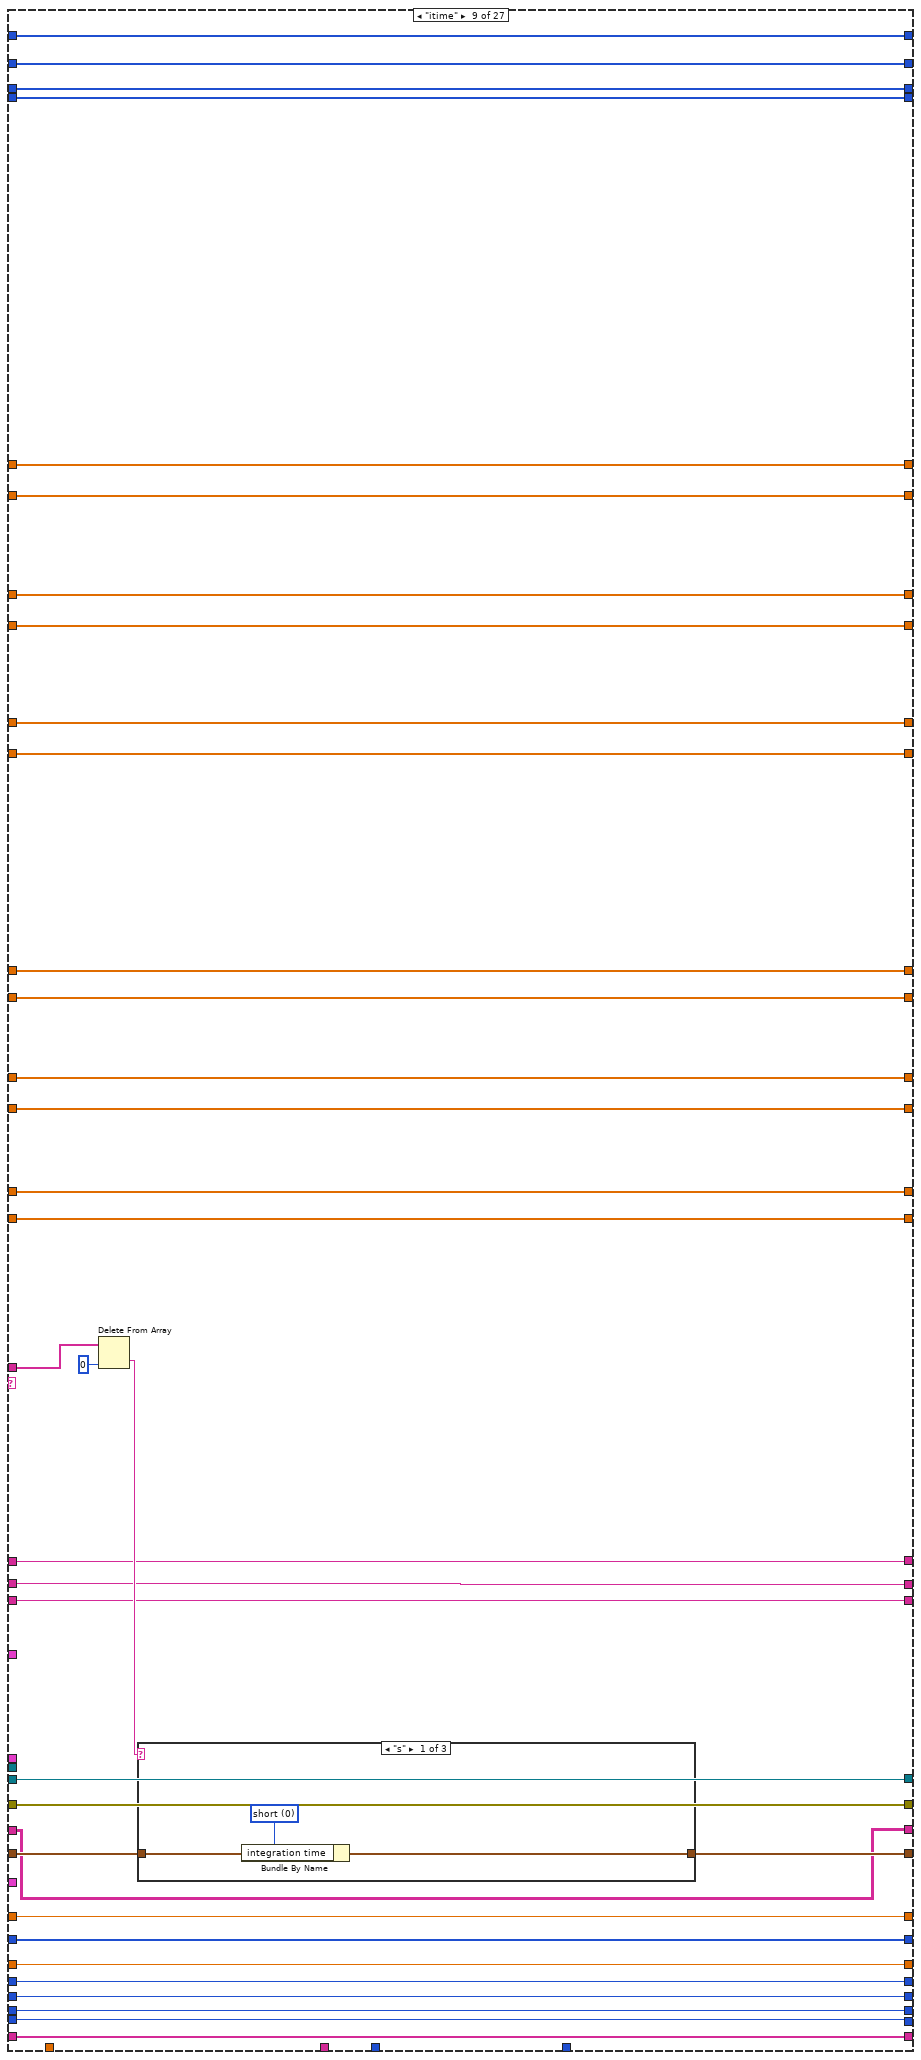
[diagram p18: hidden frame]
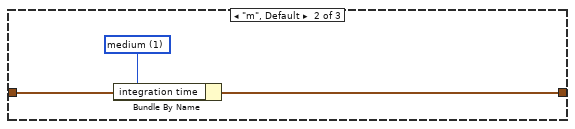
[diagram p19: hidden frame]
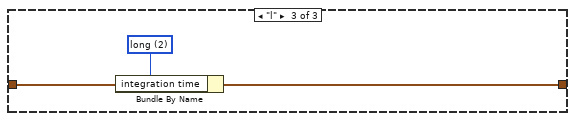
[diagram p20: hidden frame]
diagram:
  w40 = u16 1 items=["Reset All", "Partial reset"] ("Type of reset")
  # "Change from previous version:\n\n- Added a command to change part of the filename."
  # "This is a version specific to the SPM pump."
  # "I add 1 to both the \"total lines\" and the \"line running\" indicators because i and N begin from 0, and the script lines begin from 1."
  # "Bugs:\n\n- Graphs of Imax, Imin, Ion, Ioff vs time do not auto-reset between runs. To clear the data you need to restart the vi.\n\n- Do not connect the \"error\" wire of a Split block if it has unconnected terminals! It will halt the program."
  # "Array size"
  # "%s option converts a spreadsheet string to an array of strings."
  # "0: No of rows of array\n1: No of cols"
  # "Dimitrios Simatos\nv. 5.3"
  # "Changes from original textcontrol.vi:\n\n- Timestamp appears in filename.\n- (Only) transfer and output curves are plotted.\n- Communication with serial port.\n- Can execute any command, as all pattern matching functions were replaced. Previously, commands with special LabVIEW characters could not be executed.\n- Replaced write to file function with write to text file.\n- Replaced while loop with for loop.\n- Replaced 4155C \"Save File\" function and now the vi can save time-dependent variables.\n- Added clock with start time control and various units.\n- Changed filepath in which the program is saved.\n- Added a serial output log that keeps a history.\n- Tab control.\n- Addition of specialized serial read/write file for the SPM OEM pump.\n- Added halt and hard stop.\n- Imax, Imin, Ion, and Ioff are now saved for all Is, Id, and Ig."
  # "Search and replace LF with EOL"
  n1 = Equal?(x="integration time", y=u32 0) -> (x = y?=w44:bool)
  n2 = Select(t="Integration time (short)", s=w44, f="Integration time (long)") -> (s? t:f=w48:dbl)
  n3 = call "4155C Get Filename.vi"("error in (no error)"=errorcluster {"status"=FALSE, "code"=0, "source"=""}) -> ("error out"=w35:errorcluster, "path"=w10:path)  [unwired: 2 in, 1 out]
  "Path" <- w10
  n4 = Bundle By Name(cluster="Timings 2", "integration time"="integration time", "Short/Long integration time"=w48, "hold time (sec)"="hold time /s", "delay time (sec)"="delay time /s", "Step Time (0 disables)"="Step delay /s") -> (w33:T6)
  n5 = Path To String(path=w10) -> (string=w11:string)
  n6 = Search and Replace String(replace all?=TRUE ("replace all? (F)"), input string="Script", search string="\n", replace string="\r\n") -> (result string=w23:string)  [unwired: 4 in, 3 out]
  n7 = Match Pattern(string=w11, regular expression=".txt") -> (before substring=w6:string)  [unwired: 1 in, 3 out]
  n8 = Concatenate Strings(w6, "Suffix (script)") -> (w5:string)
  n9 = call "4155C Initialise.vi"("VISA resource name in"=refnum<visa-resource-name> "GPIB0::14::INSTR", "Reset"="Full Reset", "Type of reset"=w40, "error in (no error)"=w35, "VISA Timeout Value"=u32 10000) -> ("VISA Resource Name out"=w34:refnum<visa-resource-name>, "error out"=w3:errorcluster)
  n10 = Spreadsheet String To Array(delimiter (Tab)="\r\n", format string="%s", spreadsheet string="Script", array type (2D Dbl)="") -> (array=w14:string[][])
  n11 = Array Size(array=w14) -> (size(s)=w18:i32[])
  n12 = String To Path(string=w5) -> (path=w4:path)
  n13 = Index Array(array=w18, index=0) -> (element=w16:i32)
  n14 = Write to Text File(file (use dialog)=w4, text=w23, error in=w3) -> (error out=w2:errorcluster)  [unwired: 1 in, 2 out]
  n15 = for {
    N: w16 -> [w158]
    tunnel: "SMU4" -> [w194]
    shift-left: "Source/Drain Range" -> [w199]
    shift-right: [w195] -> _
    shift-left: "Source/Drain\nRange mode" -> [w200]
    shift-right: [w196] -> _
    shift-left: "Gate Range" -> [w201]
    shift-right: [w197] -> _
    shift-left: "Gate Range\nmode" -> [w202]
    shift-right: [w198] -> _
    shift-left: "Gate: Compliance" -> [w211]
    shift-right: [w207] -> _
    shift-left: "Drain: Compliance" -> [w212]
    shift-right: [w208] -> _
    shift-left: w33 -> [w213]
    shift-right: [w209] -> _
    shift-left: w2 -> [w214]
    shift-right: [w104] -> w9
    shift-left: w34 -> [w215]
    shift-right: [w210] -> _
    shift-left: w6 -> [w216]
    shift-right: [w108] -> _
    tunnel: "Panel Controls 2" -> [w193]
    shift-right: [w66] -> _
    shift-left: _ -> [w192]
    shift-right: [w128] -> _
    shift-left: _ -> [w188]
    tunnel: w14 -> [w187] mode=indexing
    shift-right: [w65] -> _
    shift-left: _ -> [w164]
    shift-right: [w98] -> _
    shift-left: _ -> [w150]
    shift-right: [w129] -> _
    shift-left: _ -> [w145]
    shift-right: [w110] -> _
    shift-left: _ -> [w144]
    shift-right: [w143] -> _
    shift-left: _ -> [w142]
    shift-right: [w103] -> _
    shift-left: _ -> [w125]
    shift-right: [w102] -> _
    shift-left: _ -> [w109]
    shift-right: [w99] -> _
    shift-left: _ -> [w101]
    shift-right: [w59] -> _
    shift-left: _ -> [w87]
    shift-right: [w60] -> _
    shift-left: _ -> [w86]
    shift-right: [w64] -> _
    shift-left: _ -> [w75]
    shift-right: [w63] -> _
    shift-left: _ -> [w74]
    shift-right: [w57] -> _
    shift-left: _ -> [w73]
    shift-right: [w67] -> _
    shift-left: _ -> [w72]
    shift-right: [w58] -> _
    shift-left: _ -> [w71]
    shift-right: [w56] -> _
    shift-left: _ -> [w70]
    shift-right: [w62] -> _
    shift-left: _ -> [w69]
    shift-right: [w61] -> _
    shift-left: _ -> [w68]
    shift-right: [w51] -> _
    shift-left: "Filename (variable part)" -> [w50]
    i -> [w153]
    w89 = "Time (Minutes)" ("element")
    # "Filename prefix"
    # "Is off"
    # "Is on"
    # "Ig off"
    # "Ig on"
    # "Is min"
    # "Is max"
    # "Ig min"
    # "Ig max"
    # "Id min"
    # "Id max"
    # "Id off"
    # "Id on"
    # "Pump status"
    # "Filepath and name"
    # "Pump status"
    # "Limit of command arguments (array columns). Raise if needed."
    # "Serial port data (string)"
    # "Serial port data (table)"
    # "Time array for valve position"
    # "Time array for absolute plunger position"
    # "Valve position"
    # "Absolute plunger position"
    # "Serial port data"
    # "For loop counter"
    # "<-----Equivalent to the 4155C \"Write\" subvi.----->"
    # "Headers"
    # "Save transfer curves in file."
    # "Filepath and name"
    # "Save time-dependent data."
    # "Use the time offset if your measurements do not start at t=0."
    # "Time for Imax, Imin, Ion, Ioff"
    # "Rest of elements of command"
    # "First element of command\n(case select)"
    n16 = Add(x=w153, y=1) -> (x+y=→"Line running":i32)
    n17 = Add(x=w158, y=1) -> (x+y=→"Total lines":i32)
    n18 = Index Array(array=w187, index=0 ("line index")) -> (element=w182:string)
    "Command running:" <- w182
    n19 = control-ref of="Interrupt run"() -> (w206:refnum<vi>)
    n20 = Spreadsheet String To Array(delimiter (Tab)=" ", format string="%s", spreadsheet string=w182, array type (2D Dbl)=string[] []) -> (array=w180:string[])
    n21 = Delete From Array(array=w180, index=0) -> (deleted portion=w88:string, array with subset deleted=w179:string[])  [unwired: 1 in]
    n22 = call "Elapsed Time"("Reset"="Reset", "Auto Reset"="Auto Reset") -> ("Elapsed Time (s)"=w189:dbl)  [unwired: 10 in, 7 out]
    n23 = case shown="0, Default" "Units" {
      tunnel: ["_sec" "_min" "_h"] -> w190
      tunnel: [w217 w221 w224] -> w160
      tunnel: w189 -> [w217 w220 w225]
      frame 0, Default {
      }
      frame 1 {
        n24 = Divide(x=w220, y=60.0) -> (x/y=w221:dbl)
      }
      frame 2 {
        n25 = Divide(x=w225, y=3600.0) -> (x/y=w224:dbl)
      }
    }
    n26 = Add(x=w160, y="Time Offset") -> (x+y=w159:dbl)
    n27 = To Long Integer(number=w159) -> (32bit integer=w126:i32)
    "Elapsed Time" <- w126
    n28 = case shown="\"resample-fpp\"" w88 {
      tunnel: w179 -> [w262 w300 w337 w469 w493 w639 w733 w821 w878 w923 w969 w1013 w1053 w1086 _ _ w1247 w1327 _ w1430 w1493 w1554 w1643 w1724 w1763 w1833 w1887]
      tunnel: w216 -> [w257 w296 w335 w476 w558 w647 w740 w829 w867 w912 w961 w1006 w1047 w1079 w1117 w1178 w1225 w1309 w1359 w1417 w1480 w1542 w1637 w1720 w1765 w1835 w1889]
      tunnel: w215 -> [w256 w295 w326 w447 w543 w616 w709 w797 w868 w913 w962 w1007 w1048 w1080 w1122 w1180 w1253 w1333 w1363 w1436 w1499 w1560 w1649 w1678 w1769 w1839 w1891]
      tunnel: w214 -> [w255 w294 w325 w446 w542 w615 w706 w794 w869 w914 w963 w1008 w1049 w1081 w1121 w1151 w1252 w1332 w1362 w1435 w1498 w1559 w1648 w1677 w1768 w1838 w1892]
      tunnel: w213 -> [w254 w293 w334 w472 w518 w643 w736 w825 w877 w922 w960 w1005 w1046 w1078 w1120 w1175 w1216 w1301 w1368 w1410 w1473 w1535 w1636 w1719 w1770 w1840 w1894]
      tunnel: w212 -> [w253 w292 w333 w474 w556 w645 w738 w827 w876 w921 w968 w1012 w1052 w1085 w1119 w1160 w1251 w1331 w1371 w1434 w1497 w1558 w1647 w1728 w1771 w1841 w1895]
      tunnel: w211 -> [w252 w291 w332 w473 w555 w644 w737 w826 w875 w920 w967 w1011 w1051 w1084 w1118 w1161 w1226 w1310 w1370 w1418 w1481 w1543 w1638 w1721 w1773 w1842 w1897]
      tunnel: [w256 w295 w324 w471 w553 w641 w735 w823 w868 w913 w962 w1007 w1048 w1080 w1122 w1180 w1217 w1283 w1361 w1411 w1474 w1536 w1589 w1680 w1769 w1839 w1891] -> w210
      tunnel: [w255 w294 w323 w470 w552 w640 w734 w822 w869 w914 w963 w1008 w1049 w1081 w1121 w1150 w1227 w1284 w1360 w1419 w1482 w1544 w1588 w1679 w1767 w1837 w1892] -> w124
      tunnel: [w254 w293 w334 w472 w514 w643 w736 w825 w870 w915 w960 w1005 w1046 w1078 w1120 w1175 w1216 w1301 w1368 w1410 w1473 w1535 w1636 w1719 w1770 w1840 w1894] -> w209
      tunnel: [w253 w292 w333 w474 w556 w645 w738 w827 w876 w921 w968 w1012 w1052 w1085 w1119 w1160 w1251 w1331 w1371 w1434 w1497 w1558 w1647 w1728 w1771 w1841 w1895] -> w208
      tunnel: [w252 w291 w332 w473 w555 w644 w737 w826 w875 w920 w967 w1011 w1051 w1084 w1118 w1161 w1226 w1310 w1370 w1418 w1481 w1543 w1638 w1721 w1773 w1842 w1897] -> w207
      tunnel: [w257 w296 w335 w476 w558 w647 w740 w829 w867 w912 w961 w1006 w1047 w1079 w1117 w1178 w1225 w1309 w1359 w1417 w1480 w1542 w1637 w1720 w1765 w1835 w1889] -> w108
      tunnel: w206 -> [_ _ _ w478 w562 w652 w743 w833 _ _ _ _ _ _ _ _ w1222 w1306 _ w1416 w1479 w1541 w1609 w1696 _ _ _]
      tunnel: "Gate" -> [_ _ _ w456 w546 w626 w720 w808 _ _ _ _ _ _ _ _ _ _ _ _ _ _ _ _ _ _ _]
      tunnel: "Drain 2" -> [_ _ _ w455 w545 w625 w719 w807 _ _ _ _ _ _ _ _ _ _ _ _ _ _ _ _ _ _ _]
      tunnel: "Panel Controls" -> [_ _ _ _ _ w624 w718 w806 _ _ _ _ _ _ _ _ _ _ _ _ _ _ _ _ _ _ _]
      tunnel: w202 -> [w251 w290 w331 w440 w536 w609 w704 w792 w874 w919 _ w1004 w1045 w1077 w1116 w1162 w1212 w1297 w1364 w1406 w1469 w1531 w1632 w1715 w1774 w1843 w1898]
      tunnel: w201 -> [w250 w289 w330 w439 w535 w608 w703 w791 w873 w918 w966 _ w1036 w1083 w1115 w1163 w1213 w1298 w1365 w1407 w1470 w1532 w1633 w1716 w1775 w1844 w1899]
      tunnel: w200 -> [w249 w288 w329 w438 w534 w607 w702 w790 w872 w917 w965 w1010 w1050 _ w1114 w1164 w1214 w1299 w1366 w1408 w1471 w1533 w1634 w1717 w1776 w1845 w1900]
      tunnel: w199 -> [w248 w287 w328 w437 w533 w606 w705 w793 w871 w916 w964 w1009 _ w1082 w1113 w1165 w1215 w1300 w1367 w1409 w1472 w1534 w1635 w1718 w1777 w1846 w1901]
      tunnel: [w251 w290 w331 w440 w536 w609 w704 w792 w874 w919 w959 w1004 w1045 w1077 w1116 w1162 w1212 w1297 w1364 w1406 w1469 w1531 w1632 w1715 w1774 w1843 w1898] -> w198
      tunnel: [w250 w289 w330 w439 w535 w608 w703 w791 w873 w918 w966 w996 w1036 w1083 w1115 w1163 w1213 w1298 w1365 w1407 w1470 w1532 w1633 w1716 w1775 w1844 w1899] -> w197
      tunnel: [w249 w288 w329 w438 w534 w607 w702 w790 w872 w917 w965 w1010 w1050 w1076 w1114 w1164 w1214 w1299 w1366 w1408 w1471 w1533 w1634 w1717 w1776 w1845 w1900] -> w196
      tunnel: [w248 w287 w328 w437 w533 w606 w705 w793 w871 w916 w964 w1009 w1037 w1082 w1113 w1165 w1215 w1300 w1367 w1409 w1472 w1534 w1635 w1718 w1777 w1846 w1901] -> w195
      tunnel: w194 -> [_ _ _ w432 w530 _ w698 _ _ _ _ _ _ _ _ _ _ _ _ _ _ _ _ _ _ _ _]
      tunnel: w193 -> [_ _ _ w430 w529 _ _ _ _ _ _ _ _ _ _ _ _ _ _ _ _ _ _ _ _ _ _]
      tunnel: [w247 w283 w321 w358 w506 w596 w695 w779 w866 w910 w958 w995 w1035 w1075 w1112 w1146 w1204 w1262 w1358 w1395 w1462 w1525 w1586 w1673 w1766 w1836 w1906] -> w66
      tunnel: w192 -> [w247 w283 w321 w427 w506 w596 w695 w779 w866 w910 w958 w995 w1035 w1075 w1112 w1146 w1204 w1262 w1358 w1395 w1462 w1525 w1586 w1673 w1766 w1836 w1906]
      tunnel: w159 -> [_ _ _ w424 w503 w594 w692 w776 _ _ _ _ _ _ _ w1144 w1202 w1279 _ w1392 w1459 w1522 w1583 w1669 _ _ _]
      tunnel: w190 -> [_ _ _ w421 w502 w592 w691 w775 _ _ _ _ _ _ _ w1142 w1200 w1278 _ w1391 w1458 w1521 w1582 w1670 _ w1804 _]
      tunnel: w126 -> [_ _ _ w416 _ _ _ _ _ _ _ _ _ _ _ _ _ _ _ _ _ _ _ _ _ w1807 _]
      tunnel: [w246 w282 w320 w366 w505 w595 w694 w778 w865 w909 w957 w994 w1034 w1074 w1111 w1145 w1203 w1281 w1357 w1394 w1461 w1524 w1585 w1672 w1772 w1816 w1896] -> w128
      tunnel: w188 -> [w246 w282 w320 w420 w505 w595 w694 w778 w865 w909 w957 w994 w1034 w1074 w1111 w1145 w1203 w1281 w1357 w1394 w1461 w1524 w1585 w1672 w1772 w1816 w1896]
      tunnel: [w245 w281 w319 w357 w501 w591 w690 w774 w864 w908 w956 w993 w1033 w1073 w1110 w1141 w1199 w1261 w1356 w1390 w1457 w1520 w1581 w1668 w1761 w1832 w1905] -> w65
      tunnel: w164 -> [w245 w281 w319 w414 w501 w591 w690 w774 w864 w908 w956 w993 w1033 w1073 w1110 w1141 w1199 w1261 w1356 w1390 w1457 w1520 w1581 w1668 w1761 w1832 w1905]
      tunnel: [w244 w280 w318 w407 w500 w590 w680 w773 w863 w907 w955 w992 w1032 w1072 w1109 w1140 w1198 w1277 w1355 w1389 w1456 w1519 w1580 w1667 w1760 w1831 w1902] -> w98
      tunnel: w150 -> [w244 w280 w318 w407 w500 w590 w680 w773 w863 w907 w955 w992 w1032 w1072 w1109 w1140 w1198 w1277 w1355 w1389 w1456 w1519 w1580 w1667 w1759 w1805 w1902]
      tunnel: [w243 w279 w317 w406 w499 w589 w679 w772 w862 w906 w954 w991 w1031 w1071 w1108 w1139 w1197 w1276 w1354 w1388 w1455 w1518 w1579 w1666 w1745 w1818 w1916] -> w129
      tunnel: w145 -> [w243 w279 w317 w406 w499 w589 w679 w772 w862 w906 w954 w991 w1031 w1071 w1108 w1139 w1197 w1276 w1354 w1388 w1455 w1518 w1579 w1666 w1745 w1817 w1916]
      tunnel: [w242 w278 w316 w405 w498 w588 w678 w771 w861 w905 w953 w990 w1030 w1070 w1107 w1138 w1196 w1275 w1353 w1387 w1454 w1517 w1578 w1665 w1744 w1800 w1918] -> w110
      tunnel: w144 -> [w242 w278 w316 w405 w498 w588 w678 w771 w861 w905 w953 w990 w1030 w1070 w1107 w1138 w1196 w1275 w1353 w1387 w1454 w1517 w1578 w1665 w1744 w1798 w1918]
      tunnel: [w241 w277 w315 w404 w497 w587 w677 w770 w860 w904 w952 w989 w1029 w1069 w1106 w1137 w1195 w1274 w1352 w1386 w1453 w1516 w1577 w1664 w1743 w1797 w1890] -> w143
      tunnel: w142 -> [w241 w277 w315 w404 w497 w587 w677 w770 w860 w904 w952 w989 w1029 w1069 w1106 w1137 w1195 w1274 w1352 w1386 w1453 w1516 w1577 w1664 w1743 w1808 w1890]
      tunnel: w126 -> [_ _ _ _ _ _ _ _ _ _ _ _ _ _ _ _ _ _ _ _ _ _ _ _ _ w1796 _]
      tunnel: w125 -> [w240 w276 w314 w403 w496 w586 w676 w769 w859 w903 w951 w988 w1028 w1068 w1105 w1136 w1194 w1273 w1351 w1385 w1452 w1515 w1576 w1663 w1742 w1795 w1917]
      tunnel: [w240 w276 w314 w403 w496 w586 w676 w769 w859 w903 w951 w988 w1028 w1068 w1105 w1136 w1194 w1273 w1351 w1385 w1452 w1515 w1576 w1663 w1742 w1794 w1917] -> w103
      tunnel: [w239 w275 w313 w402 w495 w585 w675 w768 w858 w902 w950 w987 w1027 w1067 w1104 w1135 w1193 w1272 w1350 w1384 w1451 w1514 w1575 w1662 w1741 w1793 w1915] -> w102
      tunnel: w109 -> [w239 w275 w313 w402 w495 w585 w675 w768 w858 w902 w950 w987 w1027 w1067 w1104 w1135 w1193 w1272 w1350 w1384 w1451 w1514 w1575 w1662 w1741 w1792 w1915]
      tunnel: [w238 w274 w312 w401 w494 w584 w674 w767 w857 w901 w949 w986 w1026 w1066 w1103 w1134 w1192 w1271 w1349 w1383 w1450 w1513 w1574 w1661 w1740 w1790 w1893] -> w99
      tunnel: w101 -> [w238 w274 w312 w401 w494 w584 w674 w767 w857 w901 w949 w986 w1026 w1066 w1103 w1134 w1192 w1271 w1349 w1383 w1450 w1513 w1574 w1661 w1740 w1789 w1893]
      tunnel: [w236 w272 w310 w351 w491 w582 w672 w765 w855 w900 w948 w984 w1024 w1064 w1101 w1132 w1191 w1270 w1348 w1382 w1449 w1511 w1573 w1660 w1739 w1788 w1911] -> w59
      tunnel: w87 -> [w236 w272 w310 w397 w491 w582 w672 w765 w855 w900 w948 w984 w1024 w1064 w1101 w1132 w1191 w1270 w1348 w1382 w1449 w1511 w1573 w1660 w1739 w1788 w1911]
      tunnel: [w237 w273 w311 w352 w492 w583 w673 w766 w856 w899 w947 w985 w1025 w1065 w1102 w1133 w1190 w1269 w1347 w1381 w1448 w1512 w1572 w1659 w1738 w1787 w1912] -> w60
      tunnel: w86 -> [w237 w273 w311 w396 w492 w583 w673 w766 w856 w899 w947 w985 w1025 w1065 w1102 w1133 w1190 w1269 w1347 w1381 w1448 w1512 w1572 w1659 w1738 w1787 w1912]
      tunnel: [w229 w265 w303 w356 w488 w580 w670 w763 w848 w897 w945 w982 w1022 w1062 w1099 w1125 w1183 w1260 w1346 w1374 w1441 w1504 w1565 w1654 w1731 w1786 w1904] -> w64
      tunnel: w75 -> [w229 w265 w303 w386 w488 w580 w670 w763 w848 w897 w945 w982 w1022 w1062 w1099 w1125 w1183 w1260 w1346 w1374 w1441 w1504 w1565 w1654 w1731 w1786 w1904]
      tunnel: [w228 w264 w302 w355 w489 w581 w671 w764 w847 w898 w946 w983 w1023 w1063 w1100 w1124 w1182 w1259 w1345 w1373 w1440 w1503 w1564 w1653 w1730 w1785 w1903] -> w63
      tunnel: w74 -> [w228 w264 w302 w385 w489 w581 w671 w764 w847 w898 w946 w983 w1023 w1063 w1100 w1124 w1182 w1259 w1345 w1373 w1440 w1503 w1564 w1653 w1730 w1785 w1903]
      tunnel: [w231 w267 w305 w361 w487 w578 w668 w761 w853 w895 w943 w980 w1020 w1060 w1097 w1127 w1185 w1264 w1340 w1376 w1443 w1506 w1567 w1652 w1735 w1783 w1908] -> w57
      tunnel: w73 -> [w231 w267 w305 w382 w487 w578 w668 w761 w853 w895 w943 w980 w1020 w1060 w1097 w1127 w1185 w1264 w1340 w1376 w1443 w1506 w1567 w1652 w1735 w1783 w1908]
      tunnel: [w230 w266 w304 w359 w490 w579 w669 w762 w854 w896 w944 w981 w1021 w1061 w1098 w1126 w1184 w1263 w1339 w1375 w1442 w1505 w1566 w1651 w1734 w1784 w1907] -> w67
      tunnel: w72 -> [w230 w266 w304 w381 w490 w579 w669 w762 w854 w896 w944 w981 w1021 w1061 w1098 w1126 w1184 w1263 w1339 w1375 w1442 w1505 w1566 w1651 w1734 w1784 w1907]
      tunnel: [w233 w269 w307 w350 w486 w576 w666 w759 w851 w893 w941 w978 w1018 w1058 w1095 w1129 w1187 w1266 w1342 w1378 w1445 w1508 w1569 w1656 w1737 w1781 w1910] -> w58
      tunnel: w71 -> [w233 w269 w307 w378 w486 w576 w666 w759 w851 w893 w941 w978 w1018 w1058 w1095 w1129 w1187 w1266 w1342 w1378 w1445 w1508 w1569 w1656 w1737 w1781 w1910]
      tunnel: [w232 w268 w306 w349 w485 w577 w667 w760 w852 w894 w942 w979 w1019 w1059 w1096 w1128 w1186 w1265 w1341 w1377 w1444 w1507 w1568 w1655 w1736 w1782 w1909] -> w56
      tunnel: w70 -> [w232 w268 w306 w377 w485 w577 w667 w760 w852 w894 w942 w979 w1019 w1059 w1096 w1128 w1186 w1265 w1341 w1377 w1444 w1507 w1568 w1655 w1736 w1782 w1909]
      tunnel: [w235 w271 w309 w354 w484 w574 w664 w757 w849 w891 w939 w976 w1016 w1056 w1093 w1131 w1189 w1268 w1344 w1380 w1447 w1510 w1571 w1658 w1733 w1779 w1914] -> w62
      tunnel: w69 -> [w235 w271 w309 w374 w484 w574 w664 w757 w849 w891 w939 w976 w1016 w1056 w1093 w1131 w1189 w1268 w1344 w1380 w1447 w1510 w1571 w1658 w1733 w1779 w1914]
      tunnel: [w234 w270 w308 w353 w483 w575 w665 w758 w850 w892 w940 w977 w1017 w1057 w1094 w1130 w1188 w1267 w1343 w1379 w1446 w1509 w1570 w1657 w1732 w1780 w1913] -> w61
      tunnel: w68 -> [w234 w270 w308 w373 w483 w575 w665 w758 w850 w892 w940 w977 w1017 w1057 w1094 w1130 w1188 w1267 w1343 w1379 w1446 w1509 w1570 w1657 w1732 w1780 w1913]
      tunnel: w50 -> [w227 w263 w301 w340 w482 w573 w663 w756 w846 w890 w938 w975 w1015 w1055 w1092 w1123 w1181 w1258 w1338 w1372 w1439 w1502 w1563 w1650 w1729 w1778 _]
      tunnel: [w227 w263 w301 w340 w482 w573 w663 w756 w846 w890 w938 w975 w1015 w1055 w1092 w1123 w1181 w1258 w1338 w1372 w1439 w1502 w1563 w1650 w1729 w1778 w1886] -> w51
      frame "wait" {
        n29 = Index Array(array=w262, index=0 ("Index")) -> (element=w260:string)
        n30 = Decimal String To Number(string=w260, default (0L)=u32 0) -> (number=w259:u32)  [unwired: 1 in, 1 out]
        n31 = Wait (ms)(milliseconds to wait=w259) -> ()  [unwired: 1 out]
      }
      frame "wait-min" {
        n32 = Index Array(array=w300, index=0 ("Index")) -> (element=w298:string)
        n33 = Decimal String To Number(string=w298, default (0L)=u32 0) -> (number=w286:u32)  [unwired: 1 in, 1 out]
        n34 = Multiply(x=w286, y=u32 60000) -> (x*y=w285:u32)
        n35 = Wait (ms)(milliseconds to wait=w285) -> ()  [unwired: 1 out]
      }
      frame "standby" {
        n36 = Index Array(array=w337, index=0 ("Index")) -> (element=w327:string)
        n37 = case shown="\"off\", Default" w327 {
          tunnel: [":PAGE:SCON:STAN 0" ":PAGE:SCON:STAN 1"] -> w322
          frame "off", Default {
          }
          frame "on" {
          }
        }
        n38 = VISA Write(VISA resource name=w326, write buffer=w322, error in (no error)=w325) -> (VISA resource name out=w324:refnum<visa-resource-name>, error out=w323:errorcluster)  [unwired: 1 out]
      }
      frame "transfer" {
        # "Adjusts graph colors."
        # "Adjusts graph colors."
        # "Is off"
        # "Is on"
        # "Ion will be the middle element of the array. The calculation of the index is done only once, since Is, Id, and Ig have the same dimensions."
        # "Ig off"
        # "Ig on"
        # "Is min"
        # "Is max"
        # "Ig min"
        # "Ig max"
        # "abs(Ig)"
        # "abs(Is)"
        # "Id min"
        # "Id max"
        # "Y1: Is\nY2: Id\nY3: Ig"
        # "abs(Id)"
        # "Adjusts graph colors."
        # "Adjusts graph colors."
        # "Id off"
        # "Id on"
        # "Don't connect the error lines\nof the two Split blocks!"
        # "Adjusts graph colors."
        # "Time array"
        n39 = Delete From Array(array=w469, index=0 ("Index")) -> (deleted portion=w467:string, array with subset deleted=w466:string[])  [unwired: 1 in]
        n40 = Bundle By Name(cluster=w430, "Emergency Stop"=w478) -> (w431:T2)
        n41 = Number To Decimal String(number=w424) -> (decimal integer string=w423:string)  [unwired: 1 in]
        n42 = case shown="\"d\", Default" w467 {
          tunnel: [w480 w481] -> w465
          frame "s" {
            w480 = u16 0 items=["Single", "Double"] ("sweep mode")
          }
          frame "d", Default {
            w481 = u16 1 items=["Single", "Double"] ("sweep mode")
          }
        }
        n43 = Fract/Exp String To Number(string=w466) -> (number=w451:dbl[])  [unwired: 3 in, 1 out]
        n44 = Concatenate Strings(w476, w340, w423, w421, "_T.txt" ("Suffix (transfer)")) -> (w477:string)
        n45 = VISA Write(VISA resource name=w447, write buffer=":PAGE:CHAN:MODE SWE;" ("write buffer (\"\")"), error in (no error)=w446) -> (VISA resource name out=w444:refnum<visa-resource-name>, error out=w445:errorcluster)  [unwired: 1 out]
        n46 = String To Path(string=w477) -> (path=w475:path)
        n47 = Index Array(array=w451, index #1=0 ("Index")) -> (element #1=w464:dbl, element #2=w463:dbl, element #3=w462:dbl)  [unwired: 2 in]
        n48 = Delete From Array(array=w451, length=3 ("Length"), index=0 ("Index")) -> (array with subset deleted=w449:dbl[])  [unwired: 1 out]
        n49 = Build Array (concatenate)(w420, w416) -> (w366:i32[])
        n50 = Bundle By Name(cluster=w456, "Gate Start"=w464, "Gate Stop"=w463, "Gate Step (linear only)"=w462, "Gate Compliance"=w473, "Range mode"=w440, "Range"=w439) -> (w441:T4)
        n51 = control-ref of="Imax vs time"() -> (w395:refnum<vi>)
        n52 = control-ref of="Imin vs time"() -> (w394:refnum<vi>)
        n53 = control-ref of="Ion vs time"() -> (w363:refnum<vi>)
        n54 = control-ref of="Ioff vs time"() -> (w362:refnum<vi>)
        n55 = control-ref of="I vs Vg"() -> (w425:refnum<vi>)
        n56 = Index Array(array=w449, index #1=0 ("Index")) -> (element #1=w459:dbl, element #2=w458:dbl, element #3=w457:dbl)  [unwired: 2 in]
        n57 = call <vilib>:"compatOverwrite.vi"("overwrite (F)"=TRUE) -> ("overwrite?"=w429:T7)
        n58 = Bundle By Name(cluster=w455, "Drain Start"=w459, "Drain Stop"=w458, "Drain Step"=w457, "Drain Compliance"=w474, "Range mode"=w438, "Range"=w437) -> (w442:T5)
        n59 = call "4155C Transfer.vi"("VISA resource name in"=w444, "Gate"=w441, "Drain"=w442, "Timings"=w472, "error in (no error)"=w445, "SMU4"=w432, "sweep mode"=w465, "Panel Controls"=w431) -> ("VG"=w428:dbl[], "Outparams"=w436:T8, "VISA Resource Name out"=w471:refnum<visa-resource-name>, "IS"=w391:dbl[], "ID"=w393:dbl[], "IG"=w390:dbl[], "error out"=w417:errorcluster, "SMU4"=w433:dbl[])  [unwired: 12 in]
        n60 = Unbundle By Name(w436) -> ("V2 Step"=w435:dbl, "V2 Start"=w434:dbl, "Number of points"=w360:i32)
        n61 = Absolute Value(x=w391) -> (abs(x)=w376:dbl[])
        n62 = Absolute Value(x=w393) -> (abs(x)=w392:dbl[])
        n63 = Absolute Value(x=w390) -> (abs(x)=w379:dbl[])
        n64 = Array Size(array=w392) -> (size(s)=w400:i32)
        n65 = Divide(x=w400, y=2) -> (x/y=w343:dbl)
        n66 = Subtract(x=w343, y=1) -> (x-y=w342:dbl)
        n67 = Array Max & Min(array=w376) -> (max value=w383:dbl, min value=w384:dbl)  [unwired: 2 out]
        n68 = Array Max & Min(array=w392) -> (max value=w426:dbl, min value=w389:dbl)  [unwired: 2 out]
        n69 = Array Max & Min(array=w379) -> (max value=w388:dbl, min value=w387:dbl)  [unwired: 2 out]
        n70 = call "4155C Split array.vi"("Number of VAR2 steps"=w360, "Y2 data in"=w393, "X data in"=w428, "Y1 data in"=w391, "Y3 data in"=w390, "error in (no error)"=w417) -> ("Array of clusters"=w419:cluster{"Y data in":dbl[], "X data in":dbl[]}[], "error out"=w348:errorcluster)  [unwired: 1 in]
        n71 = Index Array(array=w376, index=w342) -> (element=w367:dbl)
        n72 = Index Array(array=w376, index=0) -> (element=w368:dbl)
        n73 = Index Array(array=w392, index=w342) -> (element=w369:dbl)
        n74 = Index Array(array=w392, index=0) -> (element=w370:dbl)
        n75 = Index Array(array=w379, index=w342) -> (element=w372:dbl)
        n76 = Index Array(array=w379, index=0) -> (element=w371:dbl)
        n77 = local write "Ig max"(w388) -> ()
        n78 = local write "Ig min"(w387) -> ()
        n79 = local write "Is max"(w383) -> ()
        n80 = local write "Is min"(w384) -> ()
        n81 = local write "Id max"(w426) -> ()
        n82 = local write "Id min"(w389) -> ()
        n83 = local write "I vs Vg"(w419) -> ()
        n84 = Build Array (concatenate)(w382, w383) -> (w361:dbl[])
        n85 = Build Array (concatenate)(w381, w384) -> (w359:dbl[])
        n86 = local write "Is off"(w368) -> ()
        n87 = local write "Is on"(w367) -> ()
        n88 = Build Array (concatenate)(w427, w426) -> (w358:dbl[])
        n89 = Build Array (concatenate)(w414, w389) -> (w357:dbl[])
        n90 = Build Array (concatenate)(w386, w388) -> (w356:dbl[])
        n91 = Build Array (concatenate)(w385, w387) -> (w355:dbl[])
        n92 = Build Array (concatenate)(w374, w367) -> (w354:dbl[])
        n93 = Build Array (concatenate)(w373, w368) -> (w353:dbl[])
        n94 = Build Array (concatenate)(w396, w369) -> (w352:dbl[])
        n95 = Build Array (concatenate)(w397, w370) -> (w351:dbl[])
        n96 = Build Array (concatenate)(w378, w372) -> (w350:dbl[])
        n97 = Build Array (concatenate)(w377, w371) -> (w349:dbl[])
        n98 = local write "Ig off"(w371) -> ()
        n99 = local write "Ig on"(w372) -> ()
        n100 = local write "Id off"(w370) -> ()
        n101 = local write "Id on"(w369) -> ()
        n102 = call "4155C Split array.vi"("Number of VAR2 steps"=w360, "Y2 data in"=w352, "X data in"=w366, "Y1 data in"=w354, "Y3 data in"=w350, "error in (no error)"=w348) -> ("Array of clusters"=w364:cluster{"Y data in":dbl[], "X data in":dbl[]}[], "error out"=w347:errorcluster)  [unwired: 1 in]
        n103 = call "4155C Split array.vi"("Number of VAR2 steps"=w360, "Y2 data in"=w351, "X data in"=w366, "Y1 data in"=w353, "Y3 data in"=w349, "error in (no error)"=w347) -> ("Array of clusters"=w365:cluster{"Y data in":dbl[], "X data in":dbl[]}[], "error out"=w346:errorcluster)  [unwired: 1 in]
        n104 = call "4155C Split array.vi"("Number of VAR2 steps"=w360, "Y2 data in"=w358, "X data in"=w366, "Y1 data in"=w361, "Y3 data in"=w356, "error in (no error)"=w346) -> ("Array of clusters"=w418:cluster{"Y data in":dbl[], "X data in":dbl[]}[], "error out"=w345:errorcluster)  [unwired: 1 in]
        n105 = call "4155C Split array.vi"("Number of VAR2 steps"=w360, "Y2 data in"=w357, "X data in"=w366, "Y1 data in"=w359, "Y3 data in"=w355, "error in (no error)"=w345) -> ("Array of clusters"=w415:cluster{"Y data in":dbl[], "X data in":dbl[]}[], "error out"=w344:errorcluster)  [unwired: 1 in]
        n106 = Open/Create/Replace File(file path (use dialog)=w475, error in=w344, operation (0:open)=w429) -> (refnum out=w412:refnum<file>, error out=w410:errorcluster)  [unwired: 3 in, 1 out]
        n107 = call "4155C Make Big 2d array.vi"("1D Var1"=w428, "1d IS"=w391, "1d ID"=w393, "1d IG"=w390, "1d SMU4"=w433, "SMU4"=w432, "VAR2 START"=w434, "Number of VAR2 steps"=w360, "VAR2 STEP"=w435, "VAR1 Name"="Vg", "Decimal places in header"=i8 1, "VAR2 Name"="Vd") -> ("Header array"=w413:string[], "Data array"=w411:dbl[][])  [unwired: 14 in]
        n108 = local write "Imax vs time"(w418) -> ()
        n109 = local write "Imin vs time"(w415) -> ()
        n110 = local write "Ion vs time"(w364) -> ()
        n111 = local write "Ioff vs time"(w365) -> ()
        n112 = call "4155C Config Chart Colours.vi"("Numeric"=w360, "XY Graph 2"=w395) -> ()  [unwired: 6 in]
        n113 = call "4155C Config Chart Colours.vi"("Numeric"=w360, "XY Graph 2"=w394) -> ()  [unwired: 6 in]
        n114 = call "4155C Config Chart Colours.vi"("Numeric"=w360, "XY Graph 2"=w363) -> ()  [unwired: 6 in]
        n115 = call "4155C Config Chart Colours.vi"("Numeric"=w360, "XY Graph 2"=w362) -> ()  [unwired: 6 in]
        n116 = call "4155C Config Chart Colours.vi"("Numeric"=w360, "XY Graph 2"=w425) -> ()  [unwired: 6 in]
        n117 = call "4155C Write array to file.vi"("Byte Stream File Refnum"=w412, "Header"=w413, "Data Array"=w411, "error in (no error)"=w410) -> ("dup refnum"=w409:refnum<file>, "error out"=w408:errorcluster)  [unwired: 1 in]
        n118 = Close File(refnum=w409, error in=w408) -> (error out=w470:errorcluster)  [unwired: 1 out]
      }
      frame "pulsedstressV" {
        w512 = 0
        n119 = Number To Decimal String(number=w503) -> (decimal integer string=w559:string)  [unwired: 1 in]
        n120 = Delete From Array(array=w493, index=0 ("Index")) -> (deleted portion=w550:string, array with subset deleted=w549:string[])  [unwired: 1 in]
        n121 = Bundle By Name(cluster=w529, "Emergency Stop"=w562) -> (w531:T2)
        n122 = VISA Write(VISA resource name=w543, write buffer=":PAGE:CHAN:MODE SWE;" ("write buffer (\"\")"), error in (no error)=w542) -> (VISA resource name out=w540:refnum<visa-resource-name>, error out=w541:errorcluster)  [unwired: 1 out]
        n123 = Concatenate Strings(w558, "-pulsedstressV-" ("Substring"), w559, w502, ".txt" ("Substring")) -> (w561:string)
        n124 = case shown="\"d\", Default" w550 {
          tunnel: [w571 w572] -> w548
          frame "s" {
            w571 = u16 0 items=["Single", "Double"] ("sweep mode")
          }
          frame "d", Default {
            w572 = u16 1 items=["Single", "Double"] ("sweep mode")
          }
        }
        n125 = Fract/Exp String To Number(string=w549) -> (number=w544:dbl[])  [unwired: 3 in, 1 out]
        n126 = String To Path(string=w561) -> (path=w557:path)
        n127 = Index Array(array=w544, index #1=0 ("Index")) -> (element #1=w521:dbl, element #2=w520:dbl, element #3=w517:dbl, element #4=w516:dbl, element #5=w515:dbl, element #6=w519:dbl)  [unwired: 5 in]
        n128 = Bundle By Name(cluster=w518, "Pulse period"=w516, "Base voltage"=w517, "Pulse width"=w515) -> (w514:T6)
        n129 = Unbundle By Name(w514) -> ("Pulse period"=w522:dbl)
        n130 = Bundle By Name(cluster=w546, "Gate Start"=w520, "Gate Stop"=w521, "Gate Step (linear only)"=0, "Gate Compliance"=w555, "Range mode"=w536, "Range"=w535) -> (w537:T4)
        n131 = call <vilib>:"compatOverwrite.vi"("overwrite (F)"=TRUE) -> ("overwrite?"=w507:T7)
        n132 = Bundle By Name(cluster=w545, "Drain Start"=w519, "Drain Stop"=w512, "Drain Step"=w512, "Drain Compliance"=w556, "Range mode"=w534, "Range"=w533) -> (w538:T5)
        n133 = call "4155C PulsedStressV.vi"("VISA resource name in"=w540, "sweep mode"=w548, "Panel Controls"=w531, "Gate"=w537, "Drain"=w538, "Timings"=w514, "error in (no error)"=w541, "SMU4"=w530) -> ("VISA Resource Name out"=w553:refnum<visa-resource-name>, "ID"=w510:dbl[], "IG"=w508:dbl[], "Outparams"=w532:T8, "error out"=w554:errorcluster)  [unwired: 3 in]
        n134 = Unbundle By Name(w532) -> ("Number of points"=w509:i32)  [unwired: 2 out]
        n135 = for {
          N: w509 -> [_]
          tunnel: [w568] -> w511 mode=indexing
          tunnel: w522 -> [w570]
          i -> [w569]
          n136 = Multiply(x=w570, y=w569) -> (x*y=w568:dbl)
        }
        n137 = Insert Into Array(array=dbl[][] [] ("Input Array"), new element=w511) -> (w523:dbl[][])  [unwired: 2 in]
        n138 = Insert Into Array(array=w523, new element=w510) -> (w528:dbl[][])  [unwired: 2 in]
        n139 = Insert Into Array(array=w528, new element=w508) -> (w527:dbl[][])  [unwired: 2 in]
        n140 = Transpose 2D Array(2D array=w527) -> (transposed array=w526:dbl[][])
        n141 = Open/Create/Replace File(file path (use dialog)=w557, error in=w554, operation (0:open)=w507) -> (refnum out=w565:refnum<file>, error out=w566:errorcluster)  [unwired: 3 in, 1 out]
        n142 = call "4155C Write array to file.vi"("Byte Stream File Refnum"=w565, "Header"=string[] ["Time /s", "Id /A", "Ig /A"], "Data Array"=w526, "error in (no error)"=w566) -> ("dup refnum"=w563:refnum<file>, "error out"=w564:errorcluster)  [unwired: 1 in]
        n143 = Close File(refnum=w563, error in=w564) -> (error out=w552:errorcluster)  [unwired: 1 out]
      }
      frame "transfer-fpp" {
        n144 = Number To Decimal String(number=w594) -> (decimal integer string=w648:string)  [unwired: 1 in]
        n145 = Bundle By Name(cluster=w624, "Emergency Stop"=w652) -> (w660:T1)
        n146 = Delete From Array(array=w639, index=0 ("Index")) -> (deleted portion=w637:string, array with subset deleted=w636:string[])  [unwired: 1 in]
        n147 = Concatenate Strings(w647, "-transferfpp-" ("Substring"), w648, w592, ".txt" ("Substring")) -> (w650:string)
        n148 = VISA Write(VISA resource name=w616, write buffer=":PAGE:CHAN:MODE SWE;" ("write buffer (\"\")"), error in (no error)=w615) -> (VISA resource name out=w613:refnum<visa-resource-name>, error out=w614:errorcluster)  [unwired: 1 out]
        n149 = case shown="\"d\", Default" w637 {
          tunnel: [w661 w662] -> w635
          frame "s" {
            w661 = u16 0 items=["Single", "Double"] ("sweep mode")
          }
          frame "d", Default {
            w662 = u16 1 items=["Single", "Double"] ("sweep mode")
          }
        }
        n150 = Fract/Exp String To Number(string=w636) -> (number=w620:dbl[])  [unwired: 3 in, 1 out]
        n151 = String To Path(string=w650) -> (path=w646:path)
        n152 = Index Array(array=w620, index #1=0 ("Index")) -> (element #1=w634:dbl, element #2=w633:dbl, element #3=w632:dbl)  [unwired: 2 in]
        n153 = Delete From Array(array=w620, length=3 ("Length"), index=0 ("Index")) -> (array with subset deleted=w618:dbl[])  [unwired: 1 out]
        n154 = Bundle By Name(cluster=w626, "Gate Start"=w634, "Gate Stop"=w633, "Gate Step (linear only)"=w632, "Gate Compliance"=w644, "Range mode"=w609, "Range"=w608) -> (w610:T4)
        n155 = Index Array(array=w618, index #1=0 ("Index")) -> (element #1=w629:dbl, element #2=w628:dbl, element #3=w627:dbl)  [unwired: 2 in]
        n156 = call <vilib>:"compatOverwrite.vi"("overwrite (F)"=TRUE) -> ("overwrite?"=w597:T7)
        n157 = Bundle By Name(cluster=w625, "Drain Start"=w629, "Drain Stop"=w628, "Drain Step"=w627, "Drain Compliance"=w645, "Range mode"=w607, "Range"=w606) -> (w611:T5)
        n158 = call "4155C Transfer-FPP.vi"("VISA resource name in"=w613, "Gate"=w610, "Drain"=w611, "Timings"=w643, "error in (no error)"=w614, "sweep mode"=w635, "Panel Controls"=w660) -> ("VG"=w651:dbl[], "Outparams"=w605:T8, "VISA Resource Name out"=w641:refnum<visa-resource-name>, "Vprobe2"=w601:dbl[], "ID"=w600:dbl[], "IG"=w599:dbl[], "Vprobe1"=w598:dbl[], "error out"=w642:errorcluster)  [unwired: 13 in]
        n159 = Unbundle By Name(w605) -> ("V2 Step"=w604:dbl, "V2 Start"=w603:dbl, "Number of points"=w602:i32)
        n160 = Open/Create/Replace File(file path (use dialog)=w646, error in=w642, operation (0:open)=w597) -> (refnum out=w657:refnum<file>, error out=w658:errorcluster)  [unwired: 3 in, 1 out]
        n161 = call "4155C Make Big 2d array FPP.vi"("1D Var1"=w651, "1d ID"=w600, "1d Vp2"=w601, "1d IG"=w599, "1d Vp1"=w598, "VAR2 START"=w603, "Number of VAR2 steps"=w602, "VAR2 STEP"=w604, "VAR1 Name"="Vg", "Decimal places in header"=i8 1, "VAR2 Name"="Vd") -> ("Header array"=w653:string[], "Data array"=w654:dbl[][])  [unwired: 15 in]
        n162 = call "4155C Write array to file.vi"("Byte Stream File Refnum"=w657, "Header"=w653, "Data Array"=w654, "error in (no error)"=w658) -> ("dup refnum"=w655:refnum<file>, "error out"=w656:errorcluster)  [unwired: 1 in]
        n163 = Close File(refnum=w655, error in=w656) -> (error out=w640:errorcluster)  [unwired: 1 out]
      }
      frame "output" {
        n164 = Number To Decimal String(number=w692) -> (decimal integer string=w741:string)  [unwired: 1 in]
        n165 = Bundle By Name(cluster=w718, "Emergency Stop"=w743) -> (w753:T1)
        n166 = Delete From Array(array=w733, index=0 ("Index")) -> (deleted portion=w731:string, array with subset deleted=w730:string[])  [unwired: 1 in]
        n167 = Concatenate Strings(w740, w663, w741, w691, "_O.txt" ("Suffix (output)")) -> (w742:string)
        n168 = VISA Write(VISA resource name=w709, write buffer=":PAGE:CHAN:MODE SWE;" ("write buffer (\"\")"), error in (no error)=w706) -> (VISA resource name out=w708:refnum<visa-resource-name>, error out=w707:errorcluster)  [unwired: 1 out]
        n169 = case shown="\"d\", Default" w731 {
          tunnel: [w754 w755] -> w729
          frame "s" {
            w754 = u16 0 items=["Single", "Double"] ("sweep mode")
          }
          frame "d", Default {
            w755 = u16 1 items=["Single", "Double"] ("sweep mode")
          }
        }
        n170 = Fract/Exp String To Number(string=w730) -> (number=w712:dbl[])  [unwired: 3 in, 1 out]
        n171 = String To Path(string=w742) -> (path=w739:path)
        n172 = Index Array(array=w712, index #1=0 ("Index")) -> (element #1=w728:dbl, element #2=w727:dbl, element #3=w726:dbl)  [unwired: 2 in]
        n173 = Delete From Array(array=w712, length=3 ("Length"), index=0 ("Index")) -> (array with subset deleted=w711:dbl[])  [unwired: 1 out]
        n174 = control-ref of="I vs Vd"() -> (w682:refnum<vi>)
        n175 = Bundle By Name(cluster=w720, "Gate Start"=w728, "Gate Stop"=w727, "Gate Step (linear only)"=w726, "Gate Compliance"=w737, "Range mode"=w704, "Range"=w703) -> (w752:T4)
        n176 = Index Array(array=w711, index #1=0 ("Index")) -> (element #1=w723:dbl, element #2=w722:dbl, element #3=w721:dbl)  [unwired: 2 in]
        n177 = call <vilib>:"compatOverwrite.vi"("overwrite (F)"=TRUE) -> ("overwrite?"=w696:T7)
        n178 = Bundle By Name(cluster=w719, "Drain Start"=w723, "Drain Stop"=w722, "Drain Step"=w721, "Drain Compliance"=w738, "Range mode"=w702, "Range"=w705) -> (w751:T5)
        n179 = call "4155C Output.vi"("VISA resource name in"=w708, "Gate"=w752, "Drain"=w751, "Timings"=w736, "error in (no error)"=w707, "SMU4"=w698, "sweep mode"=w729, "Panel controls"=w753) -> ("VD"=w689:dbl[], "Outparams"=w700:T8, "VISA Resource Name out"=w735:refnum<visa-resource-name>, "IS"=w688:dbl[], "ID"=w687:dbl[], "IG"=w686:dbl[], "error out"=w684:errorcluster, "SMU4"=w697:dbl[])  [unwired: 12 in]
        n180 = Unbundle By Name(w700) -> ("V2 Step"=w701:dbl, "V2 Start"=w699:dbl, "Number of points"=w681:i32)
        n181 = call "4155C Split array.vi"("Number of VAR2 steps"=w681, "Y2 data in"=w687, "X data in"=w689, "Y1 data in"=w688, "Y3 data in"=w686, "error in (no error)"=w684) -> ("Array of clusters"=w685:cluster{"Y data in":dbl[], "X data in":dbl[]}[], "error out"=w683:errorcluster)  [unwired: 1 in]
        n182 = local write "I vs Vd"(w685) -> ()
        n183 = call "4155C Config Chart Colours.vi"("Numeric"=w681, "XY Graph 2"=w682) -> ()  [unwired: 6 in]
        n184 = Open/Create/Replace File(file path (use dialog)=w739, error in=w683, operation (0:open)=w696) -> (refnum out=w748:refnum<file>, error out=w749:errorcluster)  [unwired: 3 in, 1 out]
        n185 = call "4155C Make Big 2d array.vi"("1D Var1"=w689, "1d IS"=w688, "1d ID"=w687, "1d IG"=w686, "1d SMU4"=w697, "SMU4"=w698, "VAR2 START"=w699, "Number of VAR2 steps"=w681, "VAR2 STEP"=w701, "VAR1 Name"="Vd", "Decimal places in header"=i8 1, "VAR2 Name"="Vg") -> ("Header array"=w744:string[], "Data array"=w745:dbl[][])  [unwired: 14 in]
        n186 = call "4155C Write array to file.vi"("Byte Stream File Refnum"=w748, "Header"=w744, "Data Array"=w745, "error in (no error)"=w749) -> ("dup refnum"=w746:refnum<file>, "error out"=w747:errorcluster)  [unwired: 1 in]
        n187 = Close File(refnum=w746, error in=w747) -> (error out=w734:errorcluster)  [unwired: 1 out]
      }
      frame "output-fpp" {
        n188 = Number To Decimal String(number=w776) -> (decimal integer string=w830:string)  [unwired: 1 in]
        n189 = Bundle By Name(cluster=w806, "Emergency Stop"=w833) -> (w843:T1)
        n190 = Delete From Array(array=w821, index=0 ("Index")) -> (deleted portion=w819:string, array with subset deleted=w818:string[])  [unwired: 1 in]
        n191 = VISA Write(VISA resource name=w797, write buffer=":PAGE:CHAN:MODE SWE;" ("write buffer (\"\")"), error in (no error)=w794) -> (VISA resource name out=w796:refnum<visa-resource-name>, error out=w795:errorcluster)  [unwired: 1 out]
        n192 = Concatenate Strings(w829, "-outputfpp-" ("Substring"), w830, w775, ".txt" ("Substring")) -> (w832:string)
        n193 = case shown="\"d\", Default" w819 {
          tunnel: [w844 w845] -> w817
          frame "s" {
            w844 = u16 0 items=["Single", "Double"] ("sweep mode")
          }
          frame "d", Default {
            w845 = u16 1 items=["Single", "Double"] ("sweep mode")
          }
        }
        n194 = Fract/Exp String To Number(string=w818) -> (number=w800:dbl[])  [unwired: 3 in, 1 out]
        n195 = String To Path(string=w832) -> (path=w828:path)
        n196 = Index Array(array=w800, index #1=0 ("Index")) -> (element #1=w816:dbl, element #2=w815:dbl, element #3=w814:dbl)  [unwired: 2 in]
        n197 = Delete From Array(array=w800, length=3 ("Length"), index=0 ("Index")) -> (array with subset deleted=w799:dbl[])  [unwired: 1 out]
        n198 = Bundle By Name(cluster=w808, "Gate Start"=w816, "Gate Stop"=w815, "Gate Step (linear only)"=w814, "Gate Compliance"=w826, "Range mode"=w792, "Range"=w791) -> (w842:T4)
        n199 = Index Array(array=w799, index #1=0 ("Index")) -> (element #1=w811:dbl, element #2=w810:dbl, element #3=w809:dbl)  [unwired: 2 in]
        n200 = call <vilib>:"compatOverwrite.vi"("overwrite (F)"=TRUE) -> ("overwrite?"=w780:T7)
        n201 = Bundle By Name(cluster=w807, "Drain Start"=w811, "Drain Stop"=w810, "Drain Step"=w809, "Drain Compliance"=w827, "Range mode"=w790, "Range"=w793) -> (w841:T5)
        n202 = call "4155C Output-FPP.vi"("VISA resource name in"=w796, "Gate"=w842, "Drain"=w841, "Timings"=w825, "error in (no error)"=w795, "sweep mode"=w817, "Panel controls"=w843) -> ("VD"=w785:dbl[], "Outparams"=w788:T8, "VISA Resource Name out"=w823:refnum<visa-resource-name>, "Vprobe2"=w784:dbl[], "ID"=w783:dbl[], "IG"=w782:dbl[], "Vprobe1"=w781:dbl[], "error out"=w824:errorcluster)  [unwired: 13 in]
        n203 = Unbundle By Name(w788) -> ("V2 Step"=w789:dbl, "V2 Start"=w787:dbl, "Number of points"=w786:i32)
        n204 = Open/Create/Replace File(file path (use dialog)=w828, error in=w824, operation (0:open)=w780) -> (refnum out=w838:refnum<file>, error out=w839:errorcluster)  [unwired: 3 in, 1 out]
        n205 = call "4155C Make Big 2d array FPP.vi"("1D Var1"=w785, "1d ID"=w783, "1d Vp2"=w784, "1d IG"=w782, "1d Vp1"=w781, "VAR2 START"=w787, "Number of VAR2 steps"=w786, "VAR2 STEP"=w789, "VAR1 Name"="Vd", "Decimal places in header"=i8 1, "VAR2 Name"="Vg") -> ("Header array"=w834:string[], "Data array"=w835:dbl[][])  [unwired: 15 in]
        n206 = call "4155C Write array to file.vi"("Byte Stream File Refnum"=w838, "Header"=w834, "Data Array"=w835, "error in (no error)"=w839) -> ("dup refnum"=w836:refnum<file>, "error out"=w837:errorcluster)  [unwired: 1 in]
        n207 = Close File(refnum=w836, error in=w837) -> (error out=w822:errorcluster)  [unwired: 1 out]
      }
      frame "itime" {
        n208 = Delete From Array(array=w878, index=0 ("Index")) -> (deleted portion=w879:string)  [unwired: 1 in, 1 out]
        n209 = case shown="\"s\"" w879 {
          tunnel: w877 -> [w883 w885 w888]
          tunnel: [w882 w884 w887] -> w870
          frame "s" {
            w881 = u32 0 items=["short  ", "medium  ", "long  "] ("integration time 2")
            n210 = Bundle By Name(cluster=w883, "integration time"=w881) -> (w882:T6)
          }
          frame "m", Default {
            w886 = u32 1 items=["short  ", "medium  ", "long  "] ("integration time 2")
            n211 = Bundle By Name(cluster=w885, "integration time"=w886) -> (w884:T6)
          }
          frame "l" {
            w889 = u32 2 items=["short  ", "medium  ", "long  "] ("integration time 2")
            n212 = Bundle By Name(cluster=w888, "integration time"=w889) -> (w887:T6)
          }
        }
      }
      frame "pulsed" {
        n213 = Delete From Array(array=w923, index=0 ("Index")) -> (deleted portion=w924:string, array with subset deleted=w911:string[])  [unwired: 1 in]
        n214 = case shown="\"on\", Default" w924 {
          tunnel: w922 -> [w934 w937]
          tunnel: [w933 w936] -> w915
          tunnel: w911 -> [w931 _]
          frame "on", Default {
            w932 = u16 1 items=["Continuous", "Pulsed"] ("sweep method")
            n215 = Fract/Exp String To Number(string=w931) -> (number=w929:dbl[])  [unwired: 3 in, 1 out]
            n216 = Index Array(array=w929, index #1=0 ("Index")) -> (element #1=w928:dbl, element #2=w927:dbl, element #3=w926:dbl)  [unwired: 2 in]
            n217 = Bundle By Name(cluster=w934, "sweep method"=w932, "Pulse period"=w928, "Base voltage"=w927, "Pulse width"=w926) -> (w933:T6)
          }
          frame "off" {
            w935 = u16 0 items=["Continuous", "Pulsed"] ("sweep method")
            n218 = Bundle By Name(cluster=w937, "sweep method"=w935) -> (w936:T6)
          }
        }
      }
      frame "gaterangemode" {
        n219 = Delete From Array(array=w969, index=0 ("Index")) -> (deleted portion=w970:string)  [unwired: 1 in, 1 out]
        n220 = case shown="\"f\"" w970 {
          tunnel: [w972 w973 w974] -> w959
          frame "a", Default {
            w972 = u16 0 items=["Auto", "Limited", "Fixed"] ("Gate Range\nmode 2")
          }
          frame "f" {
            w973 = u16 2 items=["Auto", "Limited", "Fixed"] ("Gate Range\nmode 2")
          }
          frame "l" {
            w974 = u16 1 items=["Auto", "Limited", "Fixed"] ("Gate Range\nmode 2")
          }
        }
      }
      frame "gaterange" {
        (unwired) u8 11 items=["10fA  ", "100fA  ", "1nA  ", "10nA", "100nA", "1uA", "10uA", "100uA", "1mA", "10mA", "100mA", "1A"] ("Gate Range 2")
        n221 = Delete From Array(array=w1013, index=0 ("Index")) -> (deleted portion=w1003:string)  [unwired: 1 in, 1 out]
        n222 = Scan Value(string=w1003, format string="") -> (value=w1001:dbl)  [unwired: 1 in, 1 out]
        n223 = Logarithm Base 10(1:w1001) -> (0:w1000:dbl)
        n224 = Round To Nearest(number=w1000) -> (nearest integer value=w999:dbl)
        n225 = Add(x=w999, y=11.0) -> (x+y=w997:dbl)
        n226 = To Unsigned Byte Integer(number=w997) -> (unsigned 8bit integer=w996:u8)
      }
      frame "drainrange" {
        (unwired) u8 11 items=["10fA  ", "100fA  ", "1nA  ", "10nA", "100nA", "1uA", "10uA", "100uA", "1mA", "10mA", "100mA", "1A"] ("Gate Range 2")
        n227 = Delete From Array(array=w1053, index=0 ("Index")) -> (deleted portion=w1044:string)  [unwired: 1 in, 1 out]
        n228 = Scan Value(string=w1044, format string="") -> (value=w1042:dbl)  [unwired: 1 in, 1 out]
        n229 = Logarithm Base 10(1:w1042) -> (0:w1041:dbl)
        n230 = Round To Nearest(number=w1041) -> (nearest integer value=w1040:dbl)
        n231 = Add(x=w1040, y=11.0) -> (x+y=w1038:dbl)
        n232 = To Unsigned Byte Integer(number=w1038) -> (unsigned 8bit integer=w1037:u8)
      }
      frame "drainrangemode" {
        n233 = Delete From Array(array=w1086, index=0 ("Index")) -> (deleted portion=w1087:string)  [unwired: 1 in, 1 out]
        n234 = case shown="\"f\"" w1087 {
          tunnel: [w1089 w1090 w1091] -> w1076
          frame "a", Default {
            w1089 = u16 0 items=["Auto", "Limited", "Fixed"] ("Gate Range\nmode 2")
          }
          frame "f" {
            w1090 = u16 2 items=["Auto", "Limited", "Fixed"] ("Gate Range\nmode 2")
          }
          frame "l" {
            w1091 = u16 1 items=["Auto", "Limited", "Fixed"] ("Gate Range\nmode 2")
          }
        }
      }
      frame "Error", Default {
      }
      frame "logfile" {
        n235 = Number To Decimal String(number=w1144) -> (decimal integer string=w1179:string)  [unwired: 1 in]
        n236 = Concatenate Strings(w1178, "logfile" ("Substring"), w1179, w1142, ".txt" ("Substring")) -> (w1176:string)
        n237 = String To Path(string=w1176) -> (path=w1149:path)
        n238 = Unbundle(w1175) -> ("integration time"=w1174:u32, "Short/Long integration time"=w1173:dbl, "hold time (sec)"=w1172:dbl, "delay time (sec)"=w1171:dbl, "Step Time (0 disables)"=w1170:dbl, "sweep method"=w1169:u16, "Pulse period"=w1168:dbl, "Base voltage"=w1167:dbl, "Pulse width"=w1166:dbl)
        n239 = Build Array(w1174, w1173, w1172, w1171, w1170, w1169, w1168, w1167, w1166, w1160, w1161, w1162, w1163, w1164, w1165) -> (w1153:dbl[])
        n240 = Insert Into Array(array=dbl[][] [] ("Input Array"), new element=w1153) -> (w1152:dbl[][])  [unwired: 2 in]
        n241 = call <vilib>:"compatOverwrite.vi"("overwrite (F)"=TRUE) -> ("overwrite?"=w1147:T7)
        n242 = Open/Create/Replace File(file path (use dialog)=w1149, error in=w1151, operation (0:open)=w1147) -> (refnum out=w1157:refnum<file>, error out=w1156:errorcluster)  [unwired: 3 in, 1 out]
        n243 = call "4155C Write array to file.vi"("Byte Stream File Refnum"=w1157, "Header"=string[] ["Int Time", "Short/Long Itime", "Hold time", "Delay time", "Step time", "Sweep method", "Pulse period", "Base Voltage", "Pulse width", "Drain compliance", "Gate compliance", "Gate range mode", "Gate range", "S/D range mode", "S/D range"], "Data Array"=w1152, "error in (no error)"=w1156) -> ("dup refnum"=w1159:refnum<file>, "error out"=w1158:errorcluster)  [unwired: 1 in]
        n244 = Close File(refnum=w1159, error in=w1158) -> (error out=w1150:errorcluster)  [unwired: 1 out]
      }
      frame "sample" {
        n245 = Number To Decimal String(number=w1202) -> (decimal integer string=w1250:string)  [unwired: 1 in]
        n246 = Fract/Exp String To Number(string=w1247) -> (number=w1208:dbl[])  [unwired: 3 in, 1 out]
        n247 = Concatenate Strings(w1225, "-sample-" ("Substring"), w1250, w1200, ".txt" ("Substring")) -> (w1248:string)
        n248 = Index Array(array=w1208, index=0 ("Index")) -> (element=w1245:dbl)
        n249 = String To Path(string=w1248) -> (path=w1229:path)
        n250 = Index Array(array=w1208, index=2 ("Index")) -> (element=w1241:dbl)
        n251 = Index Array(array=w1208, index=3 ("Index")) -> (element=w1210:dbl)
        n252 = Index Array(array=w1208, index=4 ("Index")) -> (element=w1207:dbl)
        n253 = call "4155C Config Sampling Measurements.vi"("Sampling interval"=w1207, "Sample time"=w1210, "Display on/off"=TRUE, "Timings"=w1216, "Num Points"=w1241, "error in (no error)"=w1252, "Drain Compliance"=w1251, "Gate Compliance"=w1226, "VISA session"=w1253) -> ("error out"=w1254:errorcluster, "dup VISA resource name"=w1255:refnum<visa-resource-name>)  [unwired: 1 in]
        n254 = Index Array(array=w1208, index=1 ("Index")) -> (element=w1242:dbl)
        n255 = call "4155C Take Sample.vi"("Emergency Stop"=w1222, "error in (no error)"=w1254, "Vd"=w1242, "Vg"=w1245, "VISA resource name in"=w1255) -> ("error out"=w1220:errorcluster, "Id"=w1257:dbl[], "Ig"=w1231:dbl[], "VISA Resource Name out"=w1218:refnum<visa-resource-name>, "Is"=w1256:dbl[], "Time"=w1235:dbl[])  [unwired: 1 in]
        n256 = Insert Into Array(array=dbl[][] [] ("Input Array"), new element=w1235) -> (w1234:dbl[][])  [unwired: 2 in]
        n257 = Insert Into Array(array=w1234, new element=w1231) -> (w1233:dbl[][])  [unwired: 2 in]
        n258 = Insert Into Array(array=w1233, new element=w1257) -> (w1232:dbl[][])  [unwired: 2 in]
        n259 = VISA Write(VISA resource name=w1218, write buffer=":DISP ON" ("write buffer (\"\")"), error in (no error)=w1220) -> (VISA resource name out=w1217:refnum<visa-resource-name>, error out=w1219:errorcluster)  [unwired: 1 out]
        n260 = Insert Into Array(array=w1232, new element=w1256) -> (w1224:dbl[][])  [unwired: 2 in]
        n261 = Transpose 2D Array(2D array=w1224) -> (transposed array=w1223:dbl[][])
        n262 = call <vilib>:"compatOverwrite.vi"("overwrite (F)"=TRUE) -> ("overwrite?"=w1205:T7)
        n263 = Open/Create/Replace File(file path (use dialog)=w1229, error in=w1219, operation (0:open)=w1205) -> (refnum out=w1238:refnum<file>, error out=w1237:errorcluster)  [unwired: 3 in, 1 out]
        n264 = call "4155C Write array to file.vi"("Byte Stream File Refnum"=w1238, "Header"=string[] ["Time /s", "Ig /A", "Id /A", "Is /A"], "Data Array"=w1223, "error in (no error)"=w1237) -> ("dup refnum"=w1240:refnum<file>, "error out"=w1239:errorcluster)  [unwired: 1 in]
        n265 = Close File(refnum=w1240, error in=w1239) -> (error out=w1227:errorcluster)  [unwired: 1 out]
      }
      frame "samplei" {
        n266 = Number To Decimal String(number=w1279) -> (decimal integer string=w1330:string)  [unwired: 1 in]
        n267 = Concatenate Strings(w1309, "-samplei-" ("Substring"), w1330, w1278, ".txt" ("Substring")) -> (w1328:string)
        n268 = Fract/Exp String To Number(string=w1327) -> (number=w1294:dbl[])  [unwired: 3 in, 1 out]
        n269 = String To Path(string=w1328) -> (path=w1312:path)
        n270 = Index Array(array=w1294, index=4 ("Index")) -> (element=w1288:dbl)
        n271 = Index Array(array=w1294, index=3 ("Index")) -> (element=w1289:dbl)
        n272 = Index Array(array=w1294, index=1 ("Index")) -> (element=w1291:dbl)
        n273 = Index Array(array=w1294, index=0 ("Index")) -> (element=w1292:dbl)
        n274 = Index Array(array=w1294, index=2 ("Index")) -> (element=w1290:dbl)
        n275 = call "4155C Config SamplingI Measurements.vi"("Sample time"=w1290, "Display on/off"=TRUE, "Timings"=w1301, "Num Points"=w1291, "error in (no error)"=w1332, "Sampling interval"=w1289, "VISA session"=w1333) -> ("error out"=w1334:errorcluster, "dup VISA resource name"=w1335:refnum<visa-resource-name>)  [unwired: 3 in]
        n276 = call "4155C Take SampleI.vi"("Emergency Stop"=w1306, "error in (no error)"=w1334, "Idg 2"=w1292, "Vdg compliance 2"=w1288, "VISA resource name in"=w1335) -> ("error out"=w1304:errorcluster, "Idg"=w1337:dbl[], "Vdg"=w1314:dbl[], "VISA Resource Name out"=w1302:refnum<visa-resource-name>, "Is"=w1336:dbl[], "Time"=w1318:dbl[])  [unwired: 1 in]
        n277 = Insert Into Array(array=dbl[][] [] ("Input Array"), new element=w1318) -> (w1317:dbl[][])  [unwired: 2 in]
        n278 = Insert Into Array(array=w1317, new element=w1314) -> (w1316:dbl[][])  [unwired: 2 in]
        n279 = Insert Into Array(array=w1316, new element=w1337) -> (w1315:dbl[][])  [unwired: 2 in]
        n280 = VISA Write(VISA resource name=w1302, write buffer=":DISP ON" ("write buffer (\"\")"), error in (no error)=w1304) -> (VISA resource name out=w1287:refnum<visa-resource-name>, error out=w1303:errorcluster)  [unwired: 1 out]
        n281 = Insert Into Array(array=w1315, new element=w1336) -> (w1308:dbl[][])  [unwired: 2 in]
        n282 = call <vilib>:"compatOverwrite.vi"("overwrite (F)"=TRUE) -> ("overwrite?"=w1282:T7)
        n283 = Open/Create/Replace File(file path (use dialog)=w1312, error in=w1303, operation (0:open)=w1282) -> (refnum out=w1321:refnum<file>, error out=w1320:errorcluster)  [unwired: 3 in, 1 out]
        n284 = Transpose 2D Array(2D array=w1308) -> (transposed array=w1307:dbl[][])
        n285 = call "4155C Write array to file.vi"("Byte Stream File Refnum"=w1321, "Header"=string[] ["Time /s", "Vdg /V", "Idg /A", "Is /A"], "Data Array"=w1307, "error in (no error)"=w1320) -> ("dup refnum"=w1323:refnum<file>, "error out"=w1322:errorcluster)  [unwired: 1 in]
        n286 = Close File(refnum=w1323, error in=w1322) -> (error out=w1285:errorcluster)  [unwired: 1 out]
        n287 = VISA Write(VISA resource name=w1287, write buffer=";:PAGE:SCON:STAN OFF;:PAGE:CHAN:VSU2:DIS;" ("write buffer (\"\")"), error in (no error)=w1285) -> (VISA resource name out=w1283:refnum<visa-resource-name>, error out=w1284:errorcluster)  [unwired: 1 out]
      }
      frame "#" {
        n288 = VISA Write(VISA resource name=w1363, write buffer=":DISP ON" ("write buffer (\"\")"), error in (no error)=w1362) -> (VISA resource name out=w1361:refnum<visa-resource-name>, error out=w1360:errorcluster)  [unwired: 1 out]
      }
      frame "stressV" {
        n289 = Number To Decimal String(number=w1392) -> (decimal integer string=w1433:string)  [unwired: 1 in]
        n290 = Concatenate Strings(w1417, "-stressV-" ("Substring"), w1433, w1391, ".txt" ("Substring")) -> (w1431:string)
        n291 = Fract/Exp String To Number(string=w1430) -> (number=w1403:dbl[])  [unwired: 3 in, 1 out]
        n292 = String To Path(string=w1431) -> (path=w1421:path)
        n293 = Index Array(array=w1403, index=3 ("Index")) -> (element=w1400:dbl)
        n294 = Index Array(array=w1403, index=1 ("Index")) -> (element=w1398:dbl)
        n295 = Index Array(array=w1403, index=0 ("Index")) -> (element=w1397:dbl)
        n296 = Index Array(array=w1403, index=4 ("Index")) -> (element=w1402:dbl)
        n297 = Index Array(array=w1403, index=2 ("Index")) -> (element=w1399:dbl)
        n298 = call "4155C Config V Stress.vi"("VISA session"=w1436, "ID compliance"=w1400, "VD"=w1398, "VG"=w1397, "IG compliance"=w1399, "error in (no error)"=w1435, "Display on/off"=TRUE) -> ("dup VISA resource name"=w1438:refnum<visa-resource-name>, "error out"=w1437:errorcluster)
        n299 = call "4155C Apply Stress.vi"("error in (no error)"=w1437, "Duration"=w1402, "Emergency Stop"=w1416, "VISA resource name in"=w1438) -> ("error out"=w1414:errorcluster, "VISA Resource Name out"=w1412:refnum<visa-resource-name>)
        n300 = VISA Write(VISA resource name=w1412, write buffer=":DISP ON" ("write buffer (\"\")"), error in (no error)=w1414) -> (VISA resource name out=w1411:refnum<visa-resource-name>, error out=w1413:errorcluster)  [unwired: 1 out]
        n301 = call <vilib>:"compatOverwrite.vi"("overwrite (F)"=TRUE) -> ("overwrite?"=w1396:T7)
        n302 = Open/Create/Replace File(file path (use dialog)=w1421, error in=w1413, operation (0:open)=w1396) -> (refnum out=w1424:refnum<file>, error out=w1423:errorcluster)  [unwired: 3 in, 1 out]
        n303 = call "4155C Write array to file.vi"("Byte Stream File Refnum"=w1424, "Header"=string[] ["V stress completed successfully", ""], "error in (no error)"=w1423) -> ("dup refnum"=w1426:refnum<file>, "error out"=w1425:errorcluster)  [unwired: 2 in]
        n304 = Close File(refnum=w1426, error in=w1425) -> (error out=w1419:errorcluster)  [unwired: 1 out]
      }
      frame "stressI" {
        n305 = Number To Decimal String(number=w1459) -> (decimal integer string=w1496:string)  [unwired: 1 in]
        n306 = Concatenate Strings(w1480, "-stressI-" ("Substring"), w1496, w1458, ".txt" ("Substring")) -> (w1494:string)
        n307 = Fract/Exp String To Number(string=w1493) -> (number=w1468:dbl[])  [unwired: 3 in, 1 out]
        n308 = Index Array(array=w1468, index=1 ("Index")) -> (element=w1464:dbl)
        n309 = Index Array(array=w1468, index=0 ("Index")) -> (element=w1465:dbl)
        n310 = call "4155C Config I Stress.vi"("VISA session"=w1499, "IDG"=w1465, "VDG compliance"=w1464, "error in (no error)"=w1498, "Display on/off"=TRUE) -> ("dup VISA resource name"=w1501:refnum<visa-resource-name>, "error out"=w1500:errorcluster)
        n311 = Index Array(array=w1468, index=2 ("Index")) -> (element=w1466:dbl)
        n312 = String To Path(string=w1494) -> (path=w1484:path)
        n313 = call "4155C Apply Stress.vi"("error in (no error)"=w1500, "Duration"=w1466, "Emergency Stop"=w1479, "VISA resource name in"=w1501) -> ("error out"=w1477:errorcluster, "VISA Resource Name out"=w1475:refnum<visa-resource-name>)
        n314 = VISA Write(VISA resource name=w1475, write buffer=":DISP ON" ("write buffer (\"\")"), error in (no error)=w1477) -> (VISA resource name out=w1474:refnum<visa-resource-name>, error out=w1476:errorcluster)  [unwired: 1 out]
        n315 = call <vilib>:"compatOverwrite.vi"("overwrite (F)"=TRUE) -> ("overwrite?"=w1463:T7)
        n316 = Open/Create/Replace File(file path (use dialog)=w1484, error in=w1476, operation (0:open)=w1463) -> (refnum out=w1487:refnum<file>, error out=w1486:errorcluster)  [unwired: 3 in, 1 out]
        n317 = call "4155C Write array to file.vi"("Byte Stream File Refnum"=w1487, "Header"=string[] ["I stress completed successfully", ""], "error in (no error)"=w1486) -> ("dup refnum"=w1489:refnum<file>, "error out"=w1488:errorcluster)  [unwired: 2 in]
        n318 = Close File(refnum=w1489, error in=w1488) -> (error out=w1482:errorcluster)  [unwired: 1 out]
      }
      frame "vsu2pulse" {
        n319 = Number To Decimal String(number=w1522) -> (decimal integer string=w1557:string)  [unwired: 1 in]
        n320 = Concatenate Strings(w1542, "-vsu2-" ("Substring"), w1557, w1521, ".txt" ("Substring")) -> (w1555:string)
        n321 = Fract/Exp String To Number(string=w1554) -> (number=w1530:dbl[])  [unwired: 3 in, 1 out]
        n322 = String To Path(string=w1555) -> (path=w1546:path)
        n323 = Index Array(array=w1530, index=1 ("Index")) -> (element=w1529:dbl)
        n324 = Index Array(array=w1530, index=0 ("Index")) -> (element=w1527:dbl)
        n325 = call "4155C Config VSU2 Stress.vi"("error in (no error)"=w1559, "VSU2"=w1527, "Display on/off"=TRUE, "VISA session"=w1560) -> ("error out"=w1561:errorcluster, "dup VISA resource name"=w1562:refnum<visa-resource-name>)
        n326 = call "4155C Apply Stress.vi"("error in (no error)"=w1561, "Duration"=w1529, "Emergency Stop"=w1541, "VISA resource name in"=w1562) -> ("error out"=w1539:errorcluster, "VISA Resource Name out"=w1537:refnum<visa-resource-name>)
        n327 = VISA Write(VISA resource name=w1537, write buffer=":DISP ON" ("write buffer (\"\")"), error in (no error)=w1539) -> (VISA resource name out=w1536:refnum<visa-resource-name>, error out=w1538:errorcluster)  [unwired: 1 out]
        n328 = call <vilib>:"compatOverwrite.vi"("overwrite (F)"=TRUE) -> ("overwrite?"=w1526:T7)
        n329 = Open/Create/Replace File(file path (use dialog)=w1546, error in=w1538, operation (0:open)=w1526) -> (refnum out=w1549:refnum<file>, error out=w1548:errorcluster)  [unwired: 3 in, 1 out]
        n330 = call "4155C Write array to file.vi"("Byte Stream File Refnum"=w1549, "Header"=string[] ["VSU2 pulse completed successfully", ""], "error in (no error)"=w1548) -> ("dup refnum"=w1551:refnum<file>, "error out"=w1550:errorcluster)  [unwired: 2 in]
        n331 = Close File(refnum=w1551, error in=w1550) -> (error out=w1544:errorcluster)  [unwired: 1 out]
      }
      frame "sample-fpp" {
        w1594 = string[] ["Time /s", "Id VgVd /A", "Ig VgVd /A", "Vp1 VgVd /V", "Vp2 VgVd /V"] ("Header")
        w1598 = "%d" ("format string")
        n332 = Number To Decimal String(number=w1583) -> (decimal integer string=w1646:string)  [unwired: 1 in]
        n333 = Fract/Exp String To Number(string=w1643) -> (number=w1631:dbl[])  [unwired: 3 in, 1 out]
        n334 = Concatenate Strings(w1637, "-samplefpp-" ("Substring"), w1646, w1582, ".txt" ("Substring")) -> (w1644:string)
        n335 = String To Path(string=w1644) -> (path=w1606:path)
        n336 = Index Array(array=w1631, index=0 ("Index")) -> (element=w1592:dbl)
        n337 = Index Array(array=w1631, index=1 ("Index")) -> (element=w1591:dbl)
        n338 = Index Array(array=w1631, index=2 ("Index")) -> (element=w1639:dbl)
        n339 = Index Array(array=w1631, index=3 ("Index")) -> (element=w1629:dbl)
        n340 = call "4155C Config Sampling Measurements FPP.vi"("VISA session"=w1649, "Num Points"=w1639, "Vg"=w1592, "Display on/off"=TRUE, "Gate Compliance"=w1638, "Drain Compliance"=w1647, "Standby"="Standby", "error in (no error)"=w1648, "Timings"=w1636, "Vd"=w1591, "Sample time"=w1629) -> ("dup VISA resource name"=w1608:refnum<visa-resource-name>, "error out"=w1607:errorcluster)  [unwired: 3 in]
        n341 = Number To Decimal String(number=w1592) -> (decimal integer string=w1618:string)  [unwired: 1 in]
        n342 = call "4155C Take Sample FPP.vi"("VISA resource name in"=w1608, "error in (no error)"=w1607, "Emergency Stop"=w1609) -> ("Time"=w1613:dbl[], "Vp1"=w1623:dbl[], "VISA Resource Name out"=w1589:refnum<visa-resource-name>, "Ig"=w1611:dbl[], "Id"=w1612:dbl[], "Vp2"=w1621:dbl[], "error out"=w1610:errorcluster)  [unwired: 10 in]
        n343 = Insert Into Array(array=dbl[][] [] ("Input Array"), new element=w1613) -> (w1627:dbl[][])  [unwired: 2 in]
        n344 = Number To Decimal String(number=w1591) -> (decimal integer string=w1616:string)  [unwired: 1 in]
        n345 = Insert Into Array(array=w1627, new element=w1612) -> (w1626:dbl[][])  [unwired: 2 in]
        n346 = Concatenate Strings("(Vg = " ("Substring"), w1618, "V, Vd = " ("Substring"), w1616, "V)" ("Substring")) -> (w1614:string)
        n347 = Insert Into Array(array=w1626, new element=w1611) -> (w1625:dbl[][])  [unwired: 2 in]
        n348 = Insert Into Array(array=w1625, new element=w1623) -> (w1622:dbl[][])  [unwired: 2 in]
        n349 = Insert Into Array(array=w1622, new element=w1621) -> (w1590:dbl[][])  [unwired: 2 in]
        n350 = Transpose 2D Array(2D array=w1590) -> (transposed array=w1620:dbl[][])
        n351 = call <vilib>:"compatOverwrite.vi"("overwrite (F)"=TRUE) -> ("overwrite?"=w1587:T7)
        n352 = Open/Create/Replace File(file path (use dialog)=w1606, error in=w1610, operation (0:open)=w1587) -> (refnum out=w1603:refnum<file>, error out=w1604:errorcluster)  [unwired: 3 in, 1 out]
        n353 = Array To Spreadsheet String(array=w1594, 3:w1598) -> (spreadsheet string=w1600:string)  [unwired: 1 in]
        n354 = Search and Replace String(replace all?=TRUE ("replace all? (F)"), input string=w1600, search string="VgVd", replace string=w1614) -> (result string=w1596:string)  [unwired: 4 in, 3 out]
        n355 = Spreadsheet String To Array(format string=w1598, spreadsheet string=w1596, array type (2D Dbl)=w1594) -> (array=w1595:string[])  [unwired: 1 in]
        n356 = call "4155C Write array to file.vi"("Byte Stream File Refnum"=w1603, "Header"=w1595, "Data Array"=w1620, "error in (no error)"=w1604) -> ("dup refnum"=w1601:refnum<file>, "error out"=w1602:errorcluster)  [unwired: 1 in]
        n357 = Close File(refnum=w1601, error in=w1602) -> (error out=w1588:errorcluster)  [unwired: 1 out]
      }
      frame "resample-fpp" {
        w1683 = string[] ["Time /s", "Id VgVd /A", "Ig VgVd /A", "Vp1 VgVd /V", "Vp2 VgVd /V"] ("Header")
        w1687 = "%d" ("format string")
        n358 = Number To Decimal String(number=w1669) -> (decimal integer string=w1727:string)  [unwired: 1 in]
        n359 = Fract/Exp String To Number(string=w1724) -> (number=w1676:dbl[])  [unwired: 3 in, 1 out]
        n360 = Concatenate Strings(w1720, "-resamplefpp-" ("Substring"), w1727, w1670, ".txt" ("Substring")) -> (w1725:string)
        n361 = String To Path(string=w1725) -> (path=w1695:path)
        n362 = Index Array(array=w1676, index=0 ("Index")) -> (element=w1682:dbl)
        n363 = Index Array(array=w1676, index=1 ("Index")) -> (element=w1681:dbl)
        n364 = Number To Decimal String(number=w1682) -> (decimal integer string=w1705:string)  [unwired: 1 in]
        n365 = call "4155C Take Sample FPP.vi"("VISA resource name in"=w1678, "error in (no error)"=w1677, "Emergency Stop"=w1696) -> ("Time"=w1700:dbl[], "Vp1"=w1710:dbl[], "VISA Resource Name out"=w1680:refnum<visa-resource-name>, "Ig"=w1698:dbl[], "Id"=w1699:dbl[], "Vp2"=w1708:dbl[], "error out"=w1697:errorcluster)  [unwired: 10 in]
        n366 = Insert Into Array(array=dbl[][] [] ("Input Array"), new element=w1700) -> (w1714:dbl[][])  [unwired: 2 in]
        n367 = Number To Decimal String(number=w1681) -> (decimal integer string=w1703:string)  [unwired: 1 in]
        n368 = Insert Into Array(array=w1714, new element=w1699) -> (w1713:dbl[][])  [unwired: 2 in]
        n369 = Concatenate Strings("(Vg = " ("Substring"), w1705, "V, Vd = " ("Substring"), w1703, "V)" ("Substring")) -> (w1701:string)
        n370 = Insert Into Array(array=w1713, new element=w1698) -> (w1712:dbl[][])  [unwired: 2 in]
        n371 = Insert Into Array(array=w1712, new element=w1710) -> (w1709:dbl[][])  [unwired: 2 in]
        n372 = Insert Into Array(array=w1709, new element=w1708) -> (w1675:dbl[][])  [unwired: 2 in]
        n373 = call <vilib>:"compatOverwrite.vi"("overwrite (F)"=TRUE) -> ("overwrite?"=w1674:T7)
        n374 = Open/Create/Replace File(file path (use dialog)=w1695, error in=w1697, operation (0:open)=w1674) -> (refnum out=w1692:refnum<file>, error out=w1693:errorcluster)  [unwired: 3 in, 1 out]
        n375 = Array To Spreadsheet String(array=w1683, 3:w1687) -> (spreadsheet string=w1689:string)  [unwired: 1 in]
        n376 = Transpose 2D Array(2D array=w1675) -> (transposed array=w1707:dbl[][])
        n377 = Search and Replace String(replace all?=TRUE ("replace all? (F)"), input string=w1689, search string="VgVd", replace string=w1701) -> (result string=w1685:string)  [unwired: 4 in, 3 out]
        n378 = Spreadsheet String To Array(format string=w1687, spreadsheet string=w1685, array type (2D Dbl)=w1683) -> (array=w1684:string[])  [unwired: 1 in]
        n379 = call "4155C Write array to file.vi"("Byte Stream File Refnum"=w1692, "Header"=w1684, "Data Array"=w1707, "error in (no error)"=w1693) -> ("dup refnum"=w1690:refnum<file>, "error out"=w1691:errorcluster)  [unwired: 1 in]
        n380 = Close File(refnum=w1690, error in=w1691) -> (error out=w1679:errorcluster)  [unwired: 1 out]
      }
      frame "serial" {
        n381 = local read "Termination char\n(0xA = '\\n' = LF)\n(0xD = '\\r' = CR)"() -> (w1755:u8)
        n382 = local read "Enable Termination\nChar (T)"() -> (w1756:bool)
        n383 = Index Array(array=w1763, index=0 ("Index")) -> (element=w1762:string)
        n384 = local read "parity"() -> (w1746:u16)
        n385 = local read "Delay before read (ms)"() -> (w1757:u32)
        n386 = local read "byte count"() -> (w1754:u32)
        n387 = local read "Timeout (ms)"() -> (w1753:u32)
        n388 = local read "VISA resource name"() -> (w1750:refnum<visa-resource-name>)
        n389 = local read "baud rate"() -> (w1749:u32)
        n390 = local read "Serial End Mode for Reads"() -> (w1748:u16)
        n391 = local read "data bits"() -> (w1747:u16)
        n392 = local read "stop bits"() -> (w1752:u16)
        n393 = local read "flow control"() -> (w1751:u16)
        n394 = call "Serial write and read v0.5.vi"("Delay before read (ms)"=w1757, "Termination char\n(0xA = '\\n' = LF)\n(0xD = '\\r' = CR)"=w1755, "Enable Termination\nChar (T)"=w1756, "parity"=w1746, "stop bits"=w1752, "string to write"=w1762, "flow control"=w1751, "byte count"=w1754, "Serial Settings:Serial End Mode for Reads"=w1748, "Timeout (ms)"=w1753, "error in (no error)"=w1768, "VISA resource name"=w1750, "baud rate"=w1749, "data bits"=w1747) -> ("Serial port output"=w1758:string, "error out"=w1767:errorcluster)
        n395 = Build Array (concatenate)(w1758, w1759) -> (w1760:string[])
      }
      frame "pump" {
        # "Time array for valve position"
        # "Time array for absolute plunger position"
        # "Valve position"
        # "Absolute plunger position"
        # "Remove \"_\""
        # "Check if hard stop is pressed."
        # "Check if halt is pressed."
        # "Check if pump is idle. Else halt."
        n396 = Index Array(array=w1833, index=0 ("Index")) -> (element=w1810:string)
        n397 = case shown="\"No error\", Default" w1808 {
          tunnel: w1810 -> [w1869 _ w1871 w1872 w1873 w1874 _ _ w1877 w1878 _]
          tunnel: [w1869 "/1H" w1871 w1872 w1873 w1874 "/1H" "/1H" w1877 w1878 "/1H"] -> w1809
          frame "No error", Default {
          }
          frame "Initialization" {
          }
          frame "Invalid command" {
          }
          frame "Invalid operand" {
          }
          frame "Device not initialized" {
          }
          frame "Internal failure" {
          }
          frame "Plunger overload" {
          }
          frame "Valve overload" {
          }
          frame "Plunger move not allowed" {
          }
          frame "A/D converter failure" {
          }
          frame "Command overflow" {
          }
        }
        n398 = local read "Hard stop pump"() -> (w1812:bool)
        n399 = local read "Halt pump"() -> (w1815:bool)
        n400 = local read "Serial End Mode for Reads"() -> (w1821:u16)
        n401 = local read "flow control"() -> (w1824:u16)
        n402 = local read "stop bits"() -> (w1825:u16)
        n403 = local read "parity"() -> (w1819:u16)
        n404 = local read "Delay before read (ms)"() -> (w1830:u32)
        n405 = local read "byte count"() -> (w1827:u32)
        n406 = local read "Timeout (ms)"() -> (w1826:u32)
        n407 = local read "VISA resource name"() -> (w1823:refnum<visa-resource-name>)
        n408 = local read "baud rate"() -> (w1822:u32)
        n409 = local read "Enable Termination\nChar (T)"() -> (w1829:bool)
        n410 = local read "Termination char\n(0xA = '\\n' = LF)\n(0xD = '\\r' = CR)"() -> (w1828:u8)
        n411 = case shown="True" w1815 {
          tunnel: [w1883 "/1H"] -> w1814
          tunnel: w1809 -> [w1883 _]
          frame False {
          }
          frame True {
            n412 = local write "Halt pump"(FALSE) -> ()
          }
        }
        n413 = case shown="True" w1812 {
          tunnel: [w1880 "/1T"] -> w1813
          tunnel: w1814 -> [w1880 _]
          frame False {
          }
          frame True {
            n414 = local write "Hard stop pump"(FALSE) -> ()
          }
        }
        n415 = local read "data bits"() -> (w1820:u16)
        n416 = String Subset(string=w1804, offset (0)=1) -> (substring=w1802:string)  [unwired: 1 in]
        n417 = call "SPM Pump v0.6.vi"("Termination char\n(0xA = '\\n' = LF)\n(0xD = '\\r' = CR)"=w1828, "Enable Termination\nChar (T)"=w1829, "Timeout (ms)"=w1826, "Serial Settings:Serial End Mode for Reads"=w1821, "byte count"=w1827, "Delay before read (ms)"=w1830, "Time <input>"=w1807, "error in (no error)"=w1838, "Serial port input"=w1813, "VISA resource name"=w1823, "parity"=w1819, "baud rate"=w1822, "stop bits"=w1825, "data bits"=w1820, "flow control"=w1824, "Time units <input>"=w1802) -> ("Input command"=w1801:string, "Serial port data"=w1791:string[], "Pump status"=w1797:string, "Valve position"=w1799:i32, "Absolute plunger position"=w1811:i32, "Serial port"=w1806:string, "error out"=w1837:errorcluster)  [unwired: 1 in, 4 out]
        n418 = case shown="\"?6\"" w1801 {
          tunnel: [w1850 w1858 w1864] -> w1818
          tunnel: w1817 -> [w1850 w1857 w1864]
          tunnel: w1811 -> [_ w1856 _]
          tunnel: w1798 -> [w1849 w1855 w1865]
          tunnel: [w1849 w1855 w1867] -> w1800
          tunnel: w1799 -> [_ _ w1866]
          tunnel: w1796 -> [_ w1854 w1862]
          tunnel: w1795 -> [w1848 w1853 w1863]
          tunnel: [w1848 w1852 w1863] -> w1794
          tunnel: [w1847 w1851 w1861] -> w1793
          tunnel: w1792 -> [w1847 w1851 w1860]
          frame "Q", Default {
          }
          frame "?" {
            n419 = Build Array (concatenate)(w1857, w1856) -> (w1858:i32[])
            n420 = Build Array (concatenate)(w1853, w1854) -> (w1852:i32[])
            n421 = call "4155C Split array.vi"("X data in"=w1852, "Y1 data in"=w1858) -> ("Array of clusters"=w1859:cluster{"Y data in":dbl[], "X data in":dbl[]}[])  [unwired: 5 in, 1 out]
            n422 = local write "Absolute plunger position vs time"(w1859) -> ()
          }
          frame "?6" {
            n423 = Build Array (concatenate)(w1865, w1866) -> (w1867:i32[])
            n424 = Build Array (concatenate)(w1860, w1862) -> (w1861:i32[])
            n425 = call "4155C Split array.vi"("X data in"=w1861, "Y1 data in"=w1867) -> ("Array of clusters"=w1868:cluster{"Y data in":dbl[], "X data in":dbl[]}[])  [unwired: 5 in, 1 out]
            n426 = local write "Valve position vs time"(w1868) -> ()
          }
        }
        n427 = Build Array (concatenate)(w1789, w1791) -> (w1790:string[][])
        n428 = Build Array (concatenate)(w1805, w1806) -> (w1831:string[])
      }
      frame "filename" {
        n429 = Index Array(array=w1887, index=0 ("Index")) -> (element=w1886:string)
      }
    }
    n430 = Build Array(w128, w57, w67, w66, w65, w64, w63, w62, w61, w60, w59, w58, w56) -> (w167:dbl[][])
    n431 = Transpose 2D Array(2D array=w167) -> (transposed array=w166:dbl[][])
    n432 = Concatenate Strings(w108, w51, "Imax_Imin_Ion_Ioff_vs_time.txt" ("Suffix (Imax,Imin,Ion,Ioff)")) -> (w177:string)
    n433 = Build Array(w89, "Is max (A)" ("VAR2 Name"), "Is min (A)" ("VAR2 Name"), "Id max (A)" ("VAR2 Name"), "Id min (A)" ("VAR2 Name"), "Ig max (A)" ("VAR2 Name"), "Ig min (A)" ("VAR2 Name"), "Is on (A)" ("VAR2 Name"), "Is off (A)" ("VAR2 Name"), "Id on (A)" ("VAR2 Name"), "Id off (A)" ("VAR2 Name"), "Ig on (A)" ("VAR2 Name"), "Ig off (A)" ("VAR2 Name")) -> (w172:string[])
    n434 = Array To Spreadsheet String(array=w166, 3:"%e" ("format string")) -> (spreadsheet string=w170:string)  [unwired: 1 in]
    n435 = Array To Spreadsheet String(array=w172, 3:"" ("format string")) -> (spreadsheet string=w171:string)  [unwired: 1 in]
    n436 = String To Path(string=w177) -> (path=w176:path)
    n437 = Build Array(w171, w170) -> (w169:string[])
    n438 = Write to Text File(file (use dialog)=w176, text=w169, error in=w124) -> (refnum out=w178:refnum<file>, error out=w168:errorcluster)  [unwired: 1 in, 1 out]
    n439 = Close File(refnum=w178, error in=w168) -> (error out=w107:errorcluster)  [unwired: 1 out]
    n440 = Build Array(w103, w129) -> (w134:i32[][])
    n441 = Build Array(w89, "Absolute plunger position" ("VAR2 Name")) -> (w137:string[])
    n442 = Transpose 2D Array(2D array=w134) -> (transposed array=w127:i32[][])
    n443 = Array To Spreadsheet String(array=w137, 3:"" ("format string")) -> (spreadsheet string=w136:string)  [unwired: 1 in]
    n444 = Array To Spreadsheet String(array=w127, 3:"%e" ("format string")) -> (spreadsheet string=w133:string)  [unwired: 1 in]
    n445 = Build Array(w136, w133) -> (w139:string[])
    n446 = Concatenate Strings(w108, w51, "plunger_vs_time.txt" ("Suffix (plunger)")) -> (w131:string)
    n447 = String To Path(string=w131) -> (path=w130:path)
    n448 = Write to Text File(file (use dialog)=w130, text=w139, error in=w107) -> (refnum out=w132:refnum<file>, error out=w141:errorcluster)  [unwired: 1 in, 1 out]
    n449 = Close File(refnum=w132, error in=w141) -> (error out=w106:errorcluster)  [unwired: 1 out]
    n450 = Concatenate Strings(w108, w51, "serial_port_output.txt" ("Suffix (serial port log)")) -> (w147:string)
    n451 = String To Path(string=w147) -> (path=w146:path)
    n452 = Build Array(w89, "Serial port input" ("VAR2 Name"), "Pump status" ("VAR2 Name"), "Serial port output: ") -> (w93:string[])
    n453 = Array To Spreadsheet String(array=w99, 3:"" ("format string")) -> (spreadsheet string=w90:string)  [unwired: 1 in]
    n454 = Array To Spreadsheet String(array=w93, 3:"" ("format string")) -> (spreadsheet string=w91:string)  [unwired: 1 in]
    n455 = Build Array(w91, w90) -> (w92:string[])
    n456 = Array To Spreadsheet String(array=w98, 3:"" ("format string")) -> (spreadsheet string=w152:string)  [unwired: 1 in]
    n457 = Write to Text File(file (use dialog)=w146, text=w92, error in=w106) -> (refnum out=w148:refnum<file>, error out=w149:errorcluster)  [unwired: 1 in, 1 out]
    n458 = Close File(refnum=w148, error in=w149) -> (error out=w105:errorcluster)  [unwired: 1 out]
    n459 = local write "Serial port data"(w152) -> ()
    n460 = Build Array(w102, w110) -> (w116:i32[][])
    n461 = Build Array(w89, "Valve position" ("VAR2 Name")) -> (w119:string[])
    n462 = Transpose 2D Array(2D array=w116) -> (transposed array=w111:i32[][])
    n463 = Array To Spreadsheet String(array=w119, 3:"" ("format string")) -> (spreadsheet string=w118:string)  [unwired: 1 in]
    n464 = Array To Spreadsheet String(array=w111, 3:"%e" ("format string")) -> (spreadsheet string=w115:string)  [unwired: 1 in]
    n465 = Build Array(w118, w115) -> (w121:string[])
    n466 = Concatenate Strings(w108, w51, "valve_port_vs_time.txt" ("Suffix (valve)")) -> (w113:string)
    n467 = String To Path(string=w113) -> (path=w112:path)
    n468 = Write to Text File(file (use dialog)=w112, text=w121, error in=w105) -> (refnum out=w114:refnum<file>, error out=w123:errorcluster)  [unwired: 1 in, 1 out]
    n469 = Close File(refnum=w114, error in=w123) -> (error out=w104:errorcluster)  [unwired: 1 out]
  }
  "error out" <- w9
